vi "Calc Calculated Values.vi"(8 "error in":errorcluster, 10 "RT - Analysis Data in":T1={"RTController Data"={"State"=enum."Idle", "APU Setup Info"={"[[Sensor Info]]"=[], "[[Calibration Info]]"=[], "[[CMM Table 106]]"=[], "[[General APU Info]]"=[], "General APU Information"={"Run Count"=0}, "[[CMM Table 106B]] "=[]}, "Testing Select"=enum."Manual", "APU Select"="<Select>", "Subtests Array"=[], "Current Subtest&Step Indices"=[], "Fuel Pressure Regulator"=0.0, "Bleed-Fuel-ECS Controls"={"Fine_RC"=FALSE, "Fine_RO"=FALSE, "Coarse_RC"=FALSE, "Coarse_RO"=FALSE, "Bleed-Fine-Knob"=0.0, "Bleed-Coarse-Knob"=0.0}, "ECS Demand Cluster"={"02.06.9265.02"=4.0}, "APU & ECU Controls"={"02.00.9485.00"=FALSE, "02.01.9485.03"=FALSE, "02.01.9485.00"=FALSE, "02.01.9485.01"=FALSE, "02.00.9485.01"=FALSE, "02.00.9485.02"=FALSE, "02.00.9485.03"=FALSE, "02.00.9485.04"=FALSE, "02.00.9485.05"=FALSE, "02.01.9485.06"=FALSE, "02.00.9485.07"=FALSE, "00.04.9265.03"=FALSE}}, "Analyzed Data Sets"=[], "Current Vals"={"Post-Analysis Data"={"Calibrated Data"={"00-00-9205 Calib"=[], "00-01-9205 Calib"=[], "01-00-9213 Calib"=[], "01-01-9213 Calib"=[], "01-02-9213 Calib"=[], "02-02-9219 Calib"=[], "02-03-9227 Calib"=[], "00-02-9234 Calib"=[], "00-03-9402 Calib"=[], "02-05-9205 Calib"=[], "02-04-9871 2DArray"=[]}, "Calculated Data"={"C.00"=0.0, "C.01"=0.0, "C.02"=0.0, "C.03"=0.0, "C.04"=0.0, "C.05"=0.0, "C.06"=0.0, "C.07"=0.0, "C.08"=0.0, "C.09"=0.0, "C.10"=0.0, "C.11"=0.0, "C.12"=0.0, "C.13"=0.0, "C.14"=0.0, "C.15"=0.0, "C.16"=0.0, "C.17"=0.0, "C.18"=0.0, "C.19"=0.0, "C.20"=0.0, "C.21"=0.0, "C.22"=0.0, "C.23"=0.0, "C.24"=0.0, "C.25"=0.0, "C.26"=0.0, "C.27"=0.0, "C.28"=0.0, "C.29"=0.0, "C.30"=0.0, "C.31"=0.0, "C.32"=0.0, "C.33"=0.0, "C.34"=0.0, "C.35"=0.0, "C.36"=0.0, "C.37"=0.0, "C.38"=0.0, "C.39"=0.0, "C.40"=0.0, "C.41"=0.0, "C.42"=0.0, "C.43"=0.0, "C.44"=0.0, "C.45"=0.0, "C.46"=0.0, "C.47"=0.0, "C.48"=0.0, "C.49"=0.0, "C.50"=0.0, "C.51"=0.0, "C.52"=0.0, "C.53"=0.0, "C.54"=0.0, "C.56"=0.0}, "Indicator Data"={"00-02-9234 Power Spectras"=[], "00-02-9234 Peak Vel (in/sec)"=[], "Interactive Mode Vals"=[]}}, "Parsed Data Arrays"={"[Parsed Tags]"=[], "[VData out]"=[], "[Whole Tags]"=[]}}, "Samples/Sec"=0.0, "User Input Vals"=[], "Watchdogs"=[], "Interactive Data"={"Confirm Pressed"=FALSE, "Stored Vals"=[]}, "Accel Sensistivity"=[0.0, 0.0, 0.0], "Cutoff Frequncies"=[{"LP Passband"=0.0, "HP Stopband"=0.0, "LP Stopband"=0.0, "HP Passband"=0.0}, {"LP Passband"=0.0, "HP Stopband"=0.0, "LP Stopband"=0.0, "HP Passband"=0.0}, {"LP Passband"=0.0, "HP Stopband"=0.0, "LP Stopband"=0.0, "HP Passband"=0.0}], "Test Information"={"APU Part Number:"="", "Model:"="", "Serial Number:"="", "Customer:"="", "Work Order:"="", "Repair Level:"=""}} {"Cutoff Frequncies"."HP Passband" min=1.0 step=1.0 format="%#.4f"; "Cutoff Frequncies"."LP Stopband" min=1.0 step=1.0 format="%#.4f"; "Cutoff Frequncies"."HP Stopband" min=1.0 step=1.0 format="%#.4f"; "Cutoff Frequncies"."LP Passband" min=1.0 step=1.0 format="%#.4f"; "RTController Data"."ECS Demand Cluster"."02.06.9265.02" min=0.5 max=9.75 step=0.25 scale=0.5..9.75; "RTController Data"."Bleed-Fuel-ECS Controls"."Bleed-Coarse-Knob" min=0.0 max=1.0 step=0.001 scale=0.0..1.0; "RTController Data"."Bleed-Fuel-ECS Controls"."Bleed-Fine-Knob" min=0.0 max=1.0 step=0.001 scale=0.0..1.0; "RTController Data"."Fuel Pressure Regulator" min=0.0 max=100.0 step=0.25 scale=4.0..20.0}, 11 "[Params with Vals]":T23[](array[typedef])) -> (0 "error out":errorcluster, 3 "Calculated Values out":T16)   [LabVIEW 2018, in "RT - Analysis.lvlib"]
doc: "Performs all calculations to get the calculated values. Default output for a calculated value without an assigned calculation is NaN."
uses:
  RT - Analysis.lvlib
  Private Controls/Param Val Cluster.ctl
  Top Level/Shared Controls/Calculated Data.ctl
  Private Controls/RT-Analysis Data.ctl
  Private Controls/RTController Data.ctl
  Top Level/Shared Controls/cRIO State.ctl
  Top Level/Shared Controls/APU Setup File.ctl
  Modules/File IO/Public Controls/General APU Info.ctl
  Modules/Controller (Host)/Public Controls/Testing Select.ctl
  Modules/Controller (Host)/Public Controls/APU Select.ctl
  Modules/Testing UI 1/Public Controls/Fuel Pressure Regulator.ctl
  Modules/Testing UI 1/Public Controls/Bleed-Fuel-ECS Controls.ctl
  Modules/Testing UI 1/Public Controls/ECS Demand Controls.ctl
  Modules/Testing UI 1/Private Controls/APU & ECU Controls.ctl
  Top Level/Shared Controls/Analyzed Data Sets.ctl
  Top Level/Shared Controls/All Data Cluster.ctl
  Top Level/Shared Controls/Acq Data.ctl
  Top Level/Shared Controls/Post-Analysis Data.ctl
  Private Controls/Parsed Data Arrays.ctl
  Top Level/Shared Controls/Parsed Tag Cluster.ctl
  Private Controls/Watchdog Settings.ctl
  Private Controls/Interactive Data.ctl
  Modules/Testing UI 3/Private Controls/Cutoff Frequency.ctl
  Modules/Controller (Host)/Public Controls/Test Information.ctl
  <vilib>/Analysis/baseanly.llb/Mean (DBL).vi
  <vilib>/dlg_ctls.llb/Space Constant.vi
  Top Level/Shared VIs/Val Change Checker.vi
  <userlib>/_OpenG.lib/array/array.llb/Index Array Elements__ogtk.vi
  <userlib>/_OpenG.lib/array/array.llb/Index 1D Array Elements (Variant)__ogtk.vi
  <userlib>/_OpenG.lib/array/array.llb/Reorder 1D Array2 (DBL)__ogtk.vi
  <vilib>/Analysis/NI_AALBase.lvlib
  RT - Error Handler/RT - Error Handler.lvlib
  Modules/Controller (Host)/Controller (Host).lvlib
  Modules/Testing UI 1/Testing UI 1.lvlib
  Modules/File IO/File IO.lvlib
  Modules/Testing UI 3/Testing UI 3.lvlib
panel:
  # "Test Information:"
  # "Highpass Cutoff Frequency"
  # "Lowpass Cutoff Frequency"
  # "GTCP331-200ER Control Panel Discrete Input Panel"
  # "Bleed Load Controls"
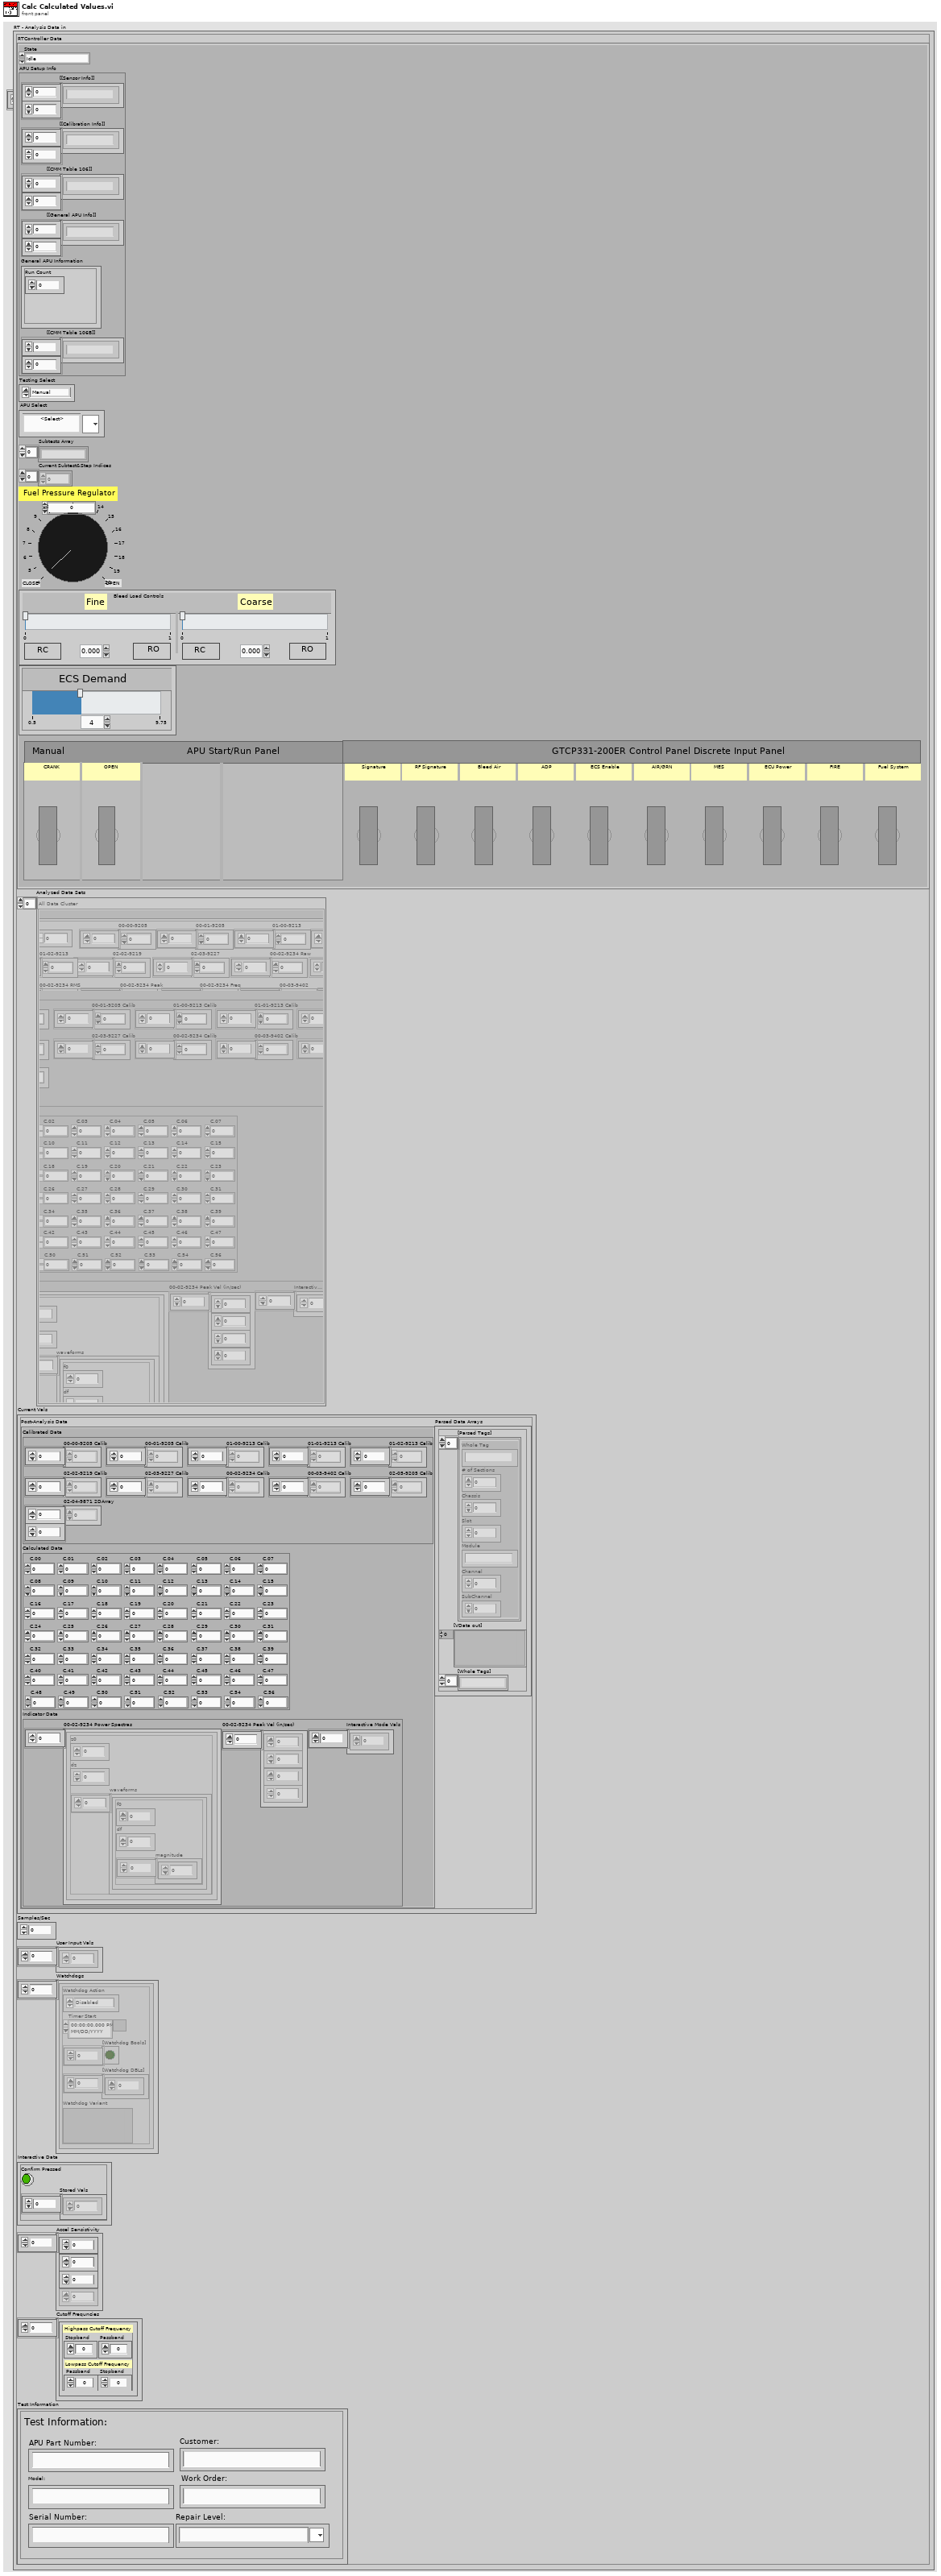
[diagram p1: front panel]
types:
  T1 = typedef "RT - Analysis.lvlib/RT-Analysis Data.ctl" = cluster{"RTController Data":T2, "Analyzed Data Sets":T12, "Current Vals":cluster{"Post-Analysis Data":T15, "Parsed Data Arrays":T17}, "Samples/Sec":dbl, "User Input Vals":dbl[], "Watchdogs":T19[], "Interactive Data":T20, "Accel Sensistivity":dbl[], "Cutoff Frequncies":T21[], "Test Information":T22}
  T2 = typedef "RT - Analysis.lvlib/RTController Data.ctl" = cluster{"State":T3, "APU Setup Info":T4, "Testing Select":T6, "APU Select":T7, "Subtests Array":string[], "Current Subtest&Step Indices":i32[], "Fuel Pressure Regulator":T8, "Bleed-Fuel-ECS Controls":T9, "ECS Demand Cluster":T10, "APU & ECU Controls":T11}
  T3 = typedef "cRIO State.ctl" = enum16{"Waiting for Cal Info", "Idle", "Calibration", "Testing"}
  T4 = typedef "APU Setup File.ctl" = cluster{"[[Sensor Info]]":string[][], "[[Calibration Info]]":string[][], "[[CMM Table 106]]":string[][], "[[General APU Info]]":string[][], "General APU Information":T5, "[[CMM Table 106B]] ":string[][]}
  T5 = typedef "File IO.lvlib/General APU Info.ctl" = cluster{"Run Count":u64}
  T6 = typedef "Controller (Host).lvlib/Testing Select.ctl" = enum16{"Manual", "Interactive", "Automatic"}
  T7 = typedef "Controller (Host).lvlib/APU Select.ctl" = string
  T8 = typedef "Testing UI 1.lvlib/Fuel Pressure Regulator.ctl" = dbl
  T9 = typedef "Testing UI 1.lvlib/Bleed-Fuel-ECS Controls.ctl" = cluster{"Fine_RC":bool, "Fine_RO":bool, "Coarse_RC":bool, "Coarse_RO":bool, "Bleed-Fine-Knob":dbl, "Bleed-Coarse-Knob":dbl}
  T10 = typedef "Testing UI 1.lvlib/ECS Demand Controls.ctl" = cluster{"02.06.9265.02":dbl}
  T11 = typedef "Testing UI 1.lvlib/APU & ECU Controls.ctl" = cluster{"02.00.9485.00":bool, "02.01.9485.03":bool, "02.01.9485.00":bool, "02.01.9485.01":bool, "02.00.9485.01":bool, "02.00.9485.02":bool, "02.00.9485.03":bool, "02.00.9485.04":bool, "02.00.9485.05":bool, "02.01.9485.06":bool, "02.00.9485.07":bool, "00.04.9265.03":bool}
  T12 = typedef "Analyzed Data Sets.ctl" = T13[]
  T13 = typedef "All Data Cluster.ctl" = cluster{"Acq Data":T14, "Post-Analysis Data":T15}
  T14 = typedef "Acq Data.ctl" = cluster{"Timestamp":timestamp, "Acq Period (ms)":i64, "00-00-9205":dbl[], "00-01-9205":dbl[], "01-00-9213":dbl[], "01-01-9213":dbl[], "01-02-9213":dbl[], "02-02-9219":dbl[], "02-03-9227":dbl[], "00-02-9234 Raw":dbl[], "00-02-9234 DC":dbl[], "00-02-9234 RMS":dbl[], "00-02-9234 Peak":dbl[], "00-02-9234 Freq":dbl[], "00-03-9402":dbl[], "02-05-9205":dbl[], "02-04-9871":dbl[]}
  T15 = typedef "Post-Analysis Data.ctl" = cluster{"Calibrated Data":cluster{"00-00-9205 Calib":dbl[], "00-01-9205 Calib":dbl[], "01-00-9213 Calib":dbl[], "01-01-9213 Calib":dbl[], "01-02-9213 Calib":dbl[], "02-02-9219 Calib":dbl[], "02-03-9227 Calib":dbl[], "00-02-9234 Calib":dbl[], "00-03-9402 Calib":dbl[], "02-05-9205 Calib":dbl[], "02-04-9871 2DArray":dbl[][]}, "Calculated Data":T16, "Indicator Data":cluster{"00-02-9234 Power Spectras":cluster{"z0":dbl, "dz":dbl, "waveforms":cluster{"f0":dbl, "df":dbl, "magnitude":dbl[]}[]}[], "00-02-9234 Peak Vel (in/sec)":dbl[], "Interactive Mode Vals":dbl[]}}
  T16 = typedef "Calculated Data.ctl" = cluster{"C.00":dbl, "C.01":dbl, "C.02":dbl, "C.03":dbl, "C.04":dbl, "C.05":dbl, "C.06":dbl, "C.07":dbl, "C.08":dbl, "C.09":dbl, "C.10":dbl, "C.11":dbl, "C.12":dbl, "C.13":dbl, "C.14":dbl, "C.15":dbl, "C.16":dbl, "C.17":dbl, "C.18":dbl, "C.19":dbl, "C.20":dbl, "C.21":dbl, "C.22":dbl, "C.23":dbl, "C.24":dbl, "C.25":dbl, "C.26":dbl, "C.27":dbl, "C.28":dbl, "C.29":dbl, "C.30":dbl, "C.31":dbl, "C.32":dbl, "C.33":dbl, "C.34":dbl, "C.35":dbl, "C.36":dbl, "C.37":dbl, "C.38":dbl, "C.39":dbl, "C.40":dbl, "C.41":dbl, "C.42":dbl, "C.43":dbl, "C.44":dbl, "C.45":dbl, "C.46":dbl, "C.47":dbl, "C.48":dbl, "C.49":dbl, "C.50":dbl, "C.51":dbl, "C.52":dbl, "C.53":dbl, "C.54":dbl, "C.56":dbl}
  T17 = typedef "RT - Analysis.lvlib/Parsed Data Arrays.ctl" = cluster{"[Parsed Tags]":T18[], "[VData out]":variant[], "[Whole Tags]":string[]}
  T18 = typedef "Parsed Tag Cluster.ctl" = cluster{"Whole Tag":string, "# of Sections":u8, "Chassis":u8, "Slot":u8, "Module":string, "Channel":u8, "SubChannel":u8}
  T19 = typedef "RT - Analysis.lvlib/Watchdog Settings.ctl" = cluster{"Watchdog Action":enum16{"Disabled", "Timer - Change Sample Rate", "RPM Thresh - Insert Other", "RPM Thresh - Check POPD", "RPM Thresh - StartStop Logging"}, "Timer Start":timestamp, "[Watchdog Bools]":bool[], "[Watchdog DBLs]":dbl[], "Watchdog Variant":variant}
  T20 = typedef "RT - Analysis.lvlib/Interactive Data.ctl" = cluster{"Confirm Pressed":bool, "Stored Vals":dbl[]}
  T21 = typedef "Testing UI 3.lvlib/Cutoff Frequency.ctl" = cluster{"LP Passband":dbl, "HP Stopband":dbl, "LP Stopband":dbl, "HP Passband":dbl}
  T22 = typedef "Controller (Host).lvlib/Test Information.ctl" = cluster{"APU Part Number:":string, "Model:":string, "Serial Number:":string, "Customer:":string, "Work Order:":string, "Repair Level:":string}
  T23 = typedef "RT - Analysis.lvlib/Param Val Cluster.ctl" = cluster{"Param":string, "Value":variant}
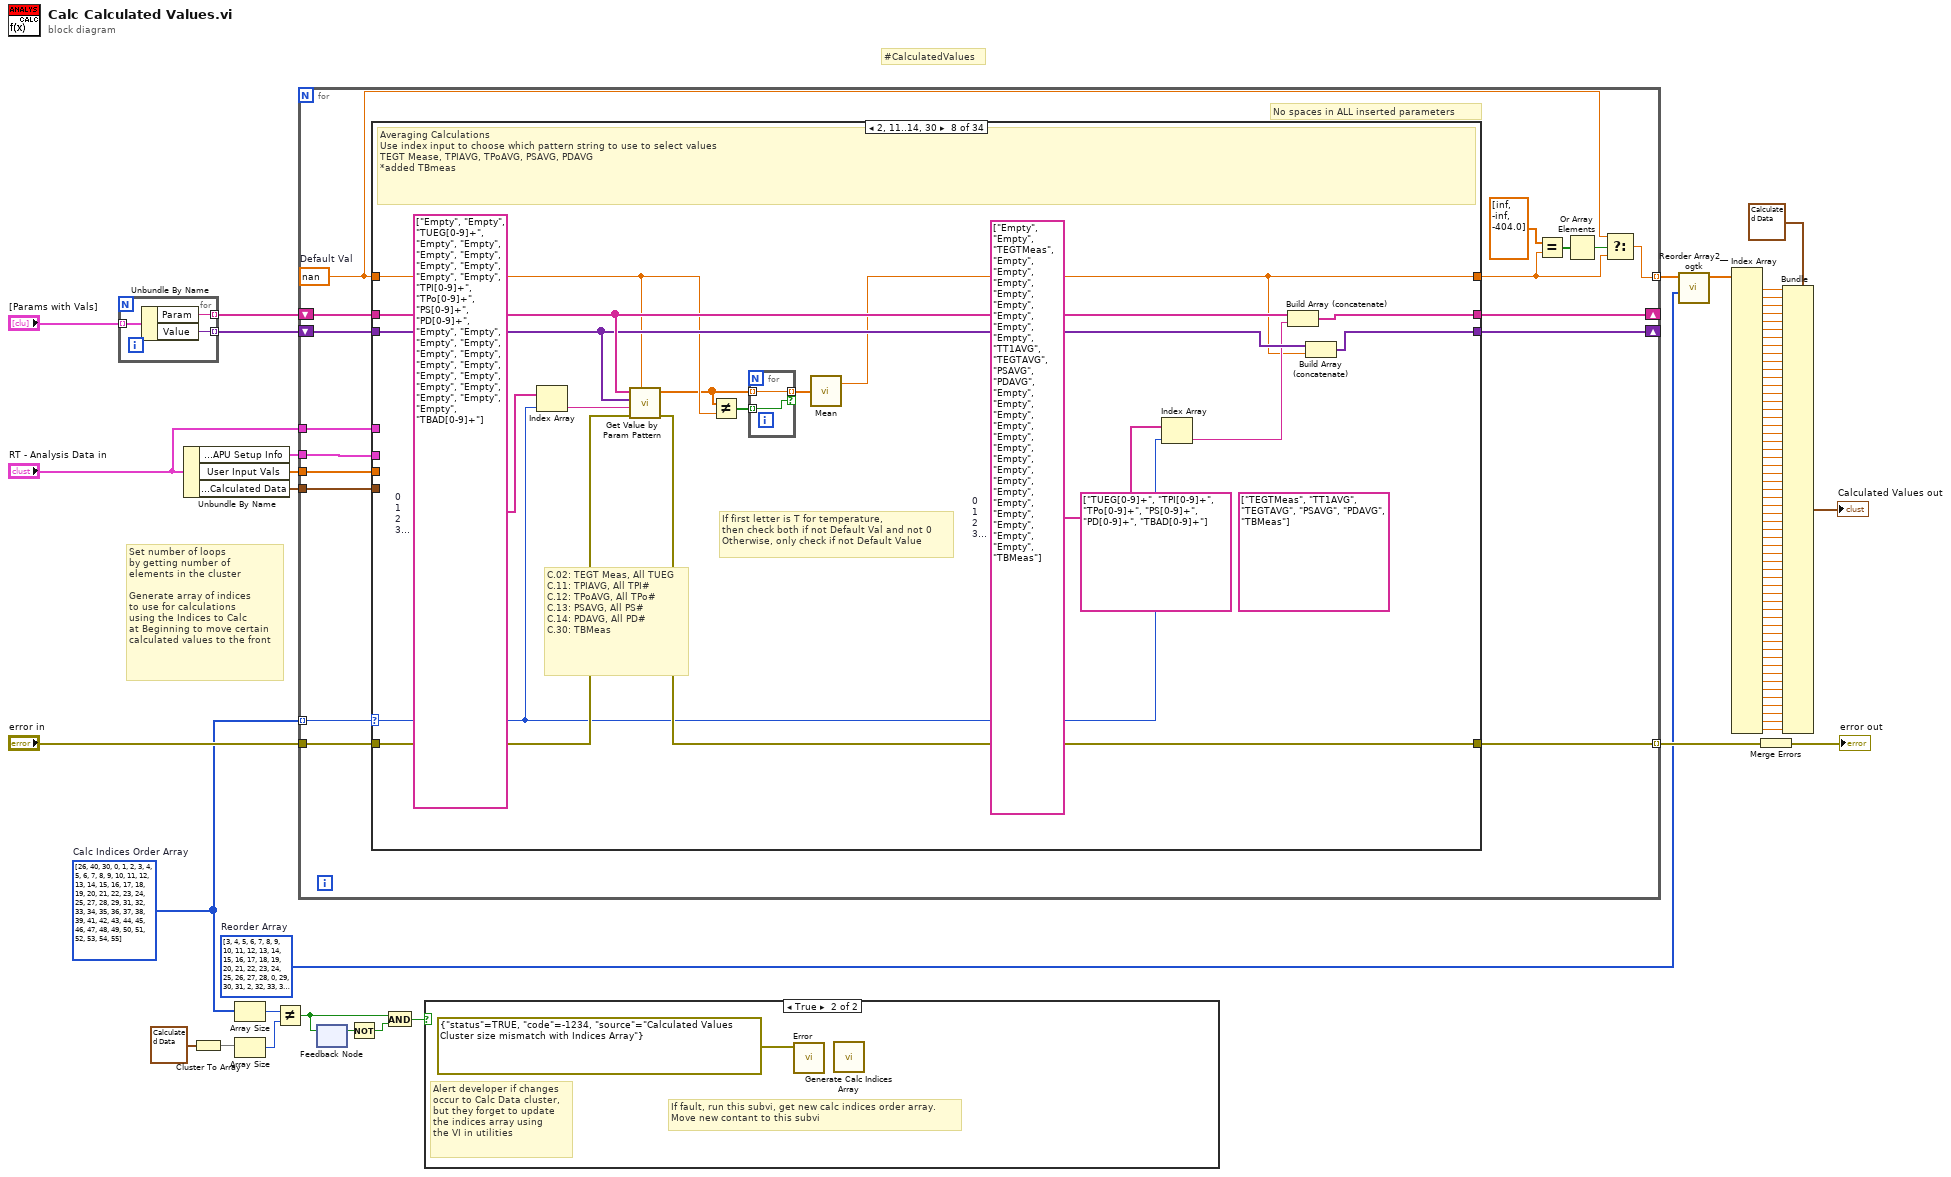
[diagram p0: block diagram]
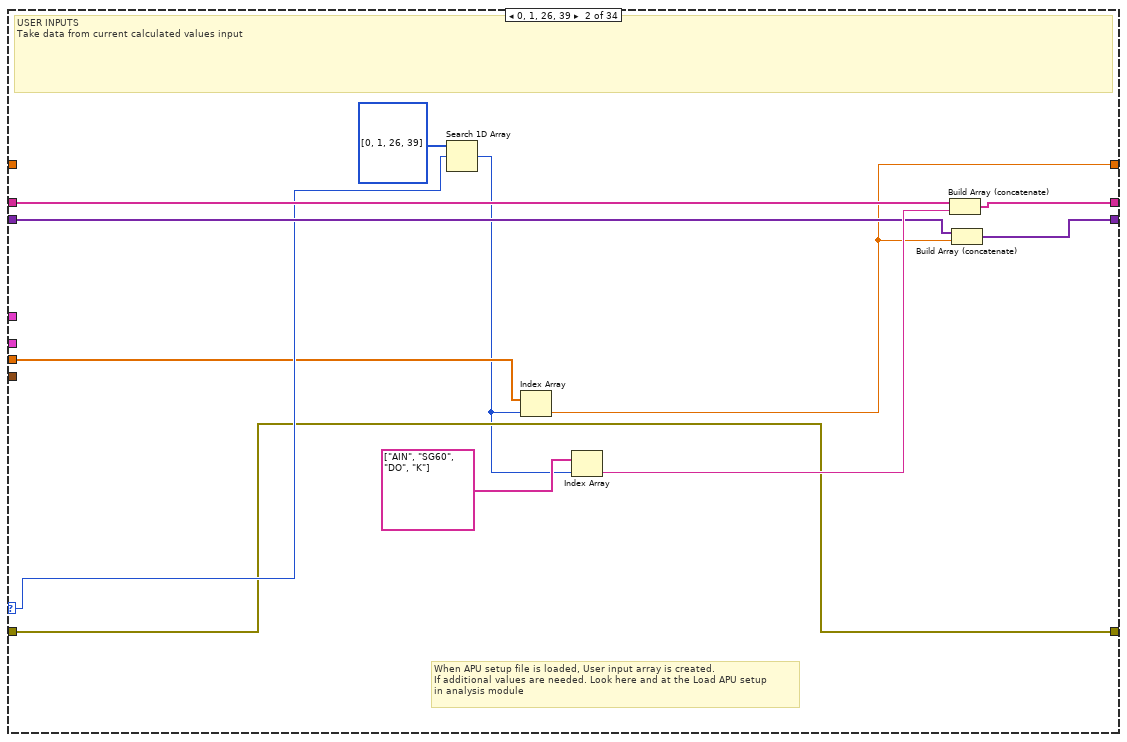
[diagram p4: hidden frame]
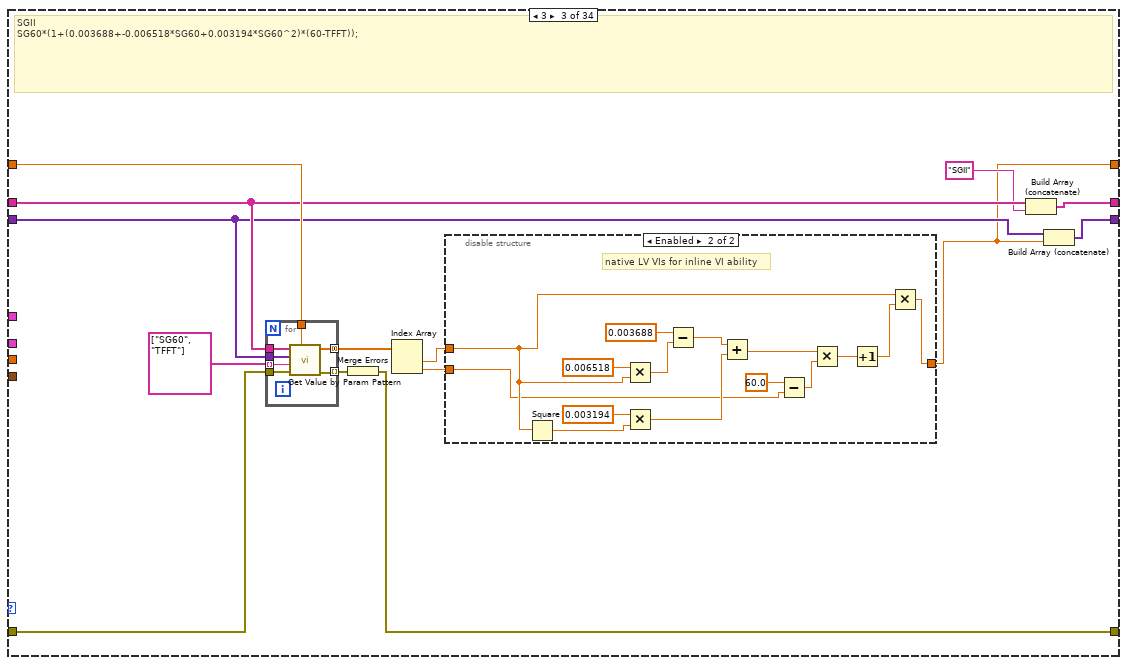
[diagram p5: hidden frame]
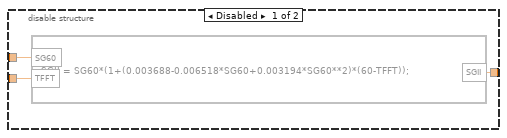
[diagram p6: hidden frame]
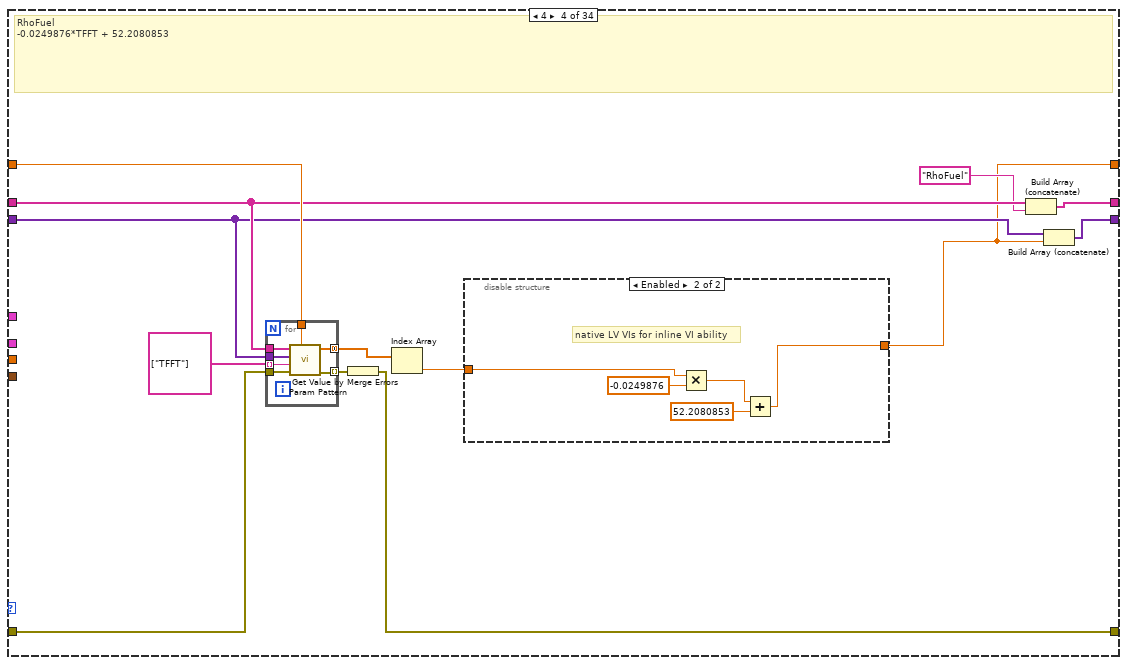
[diagram p7: hidden frame]
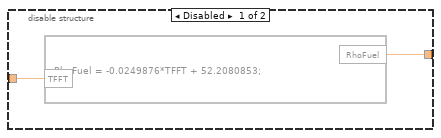
[diagram p8: hidden frame]
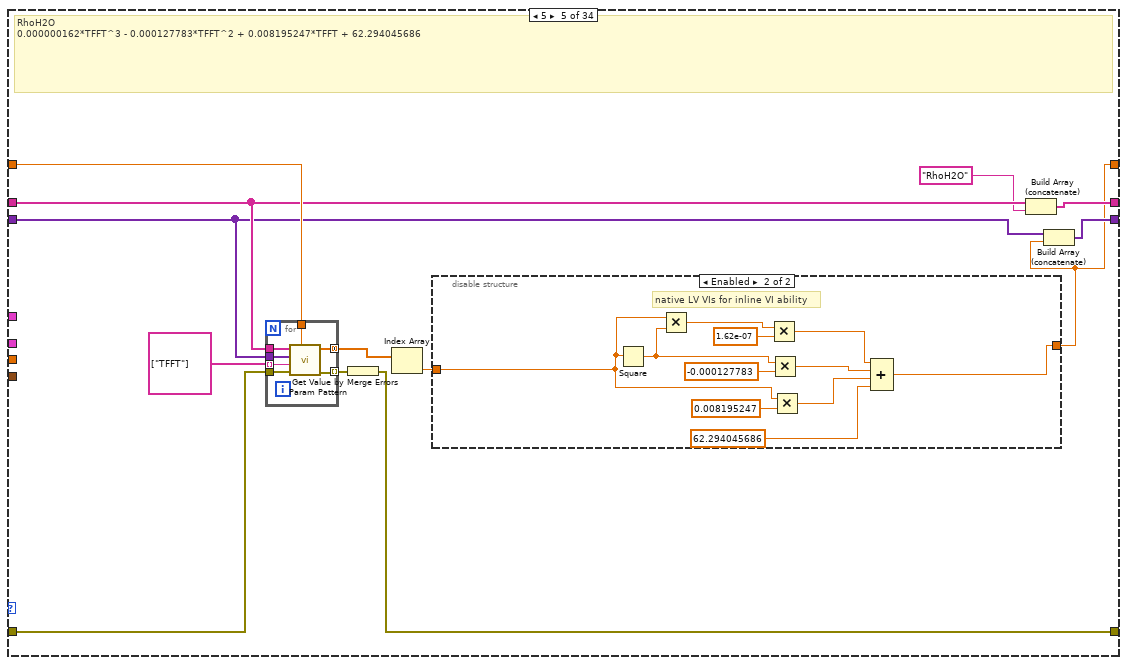
[diagram p9: hidden frame]
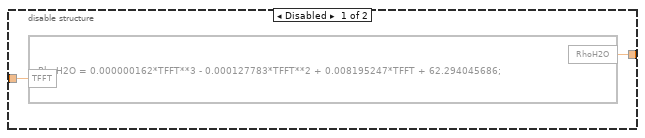
[diagram p10: hidden frame]
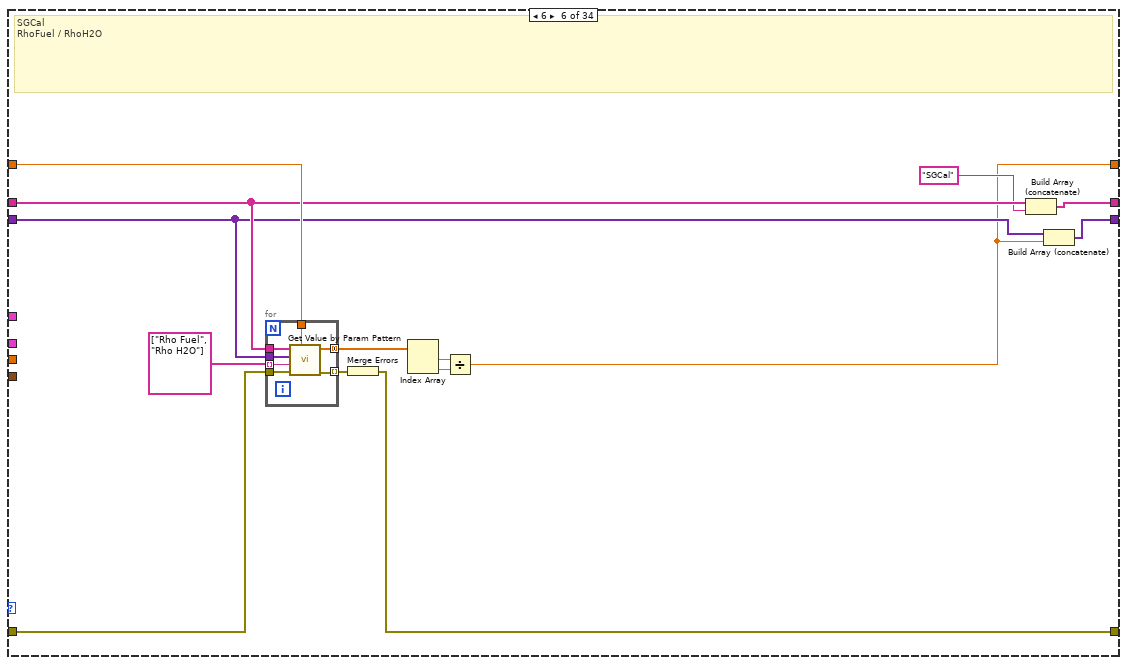
[diagram p11: hidden frame]
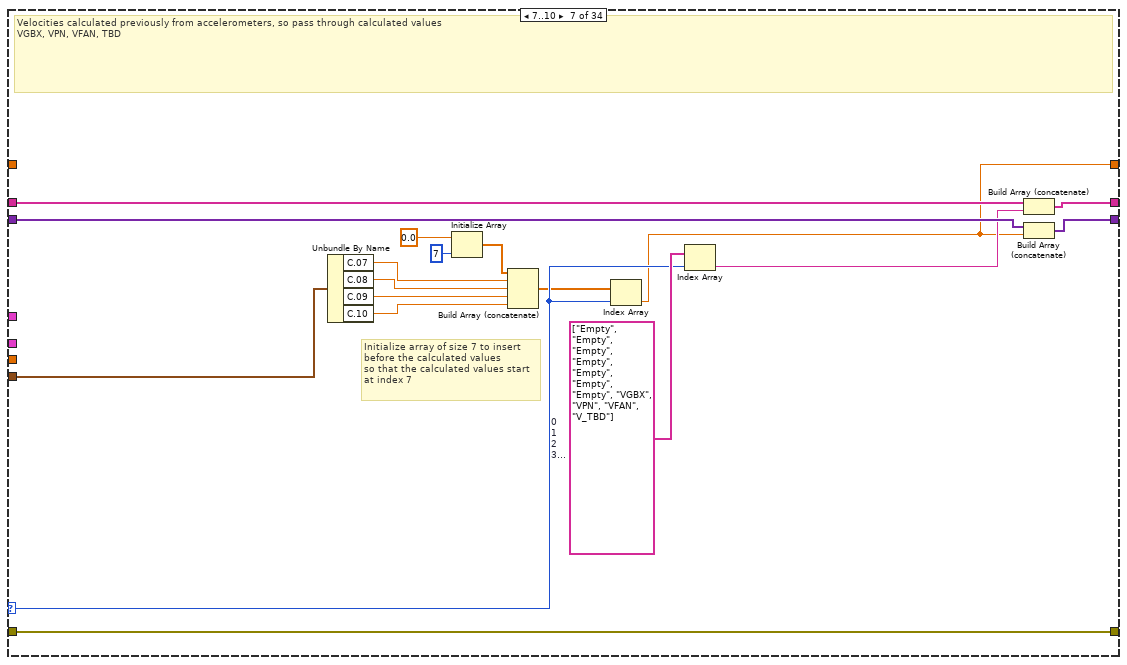
[diagram p12: hidden frame]
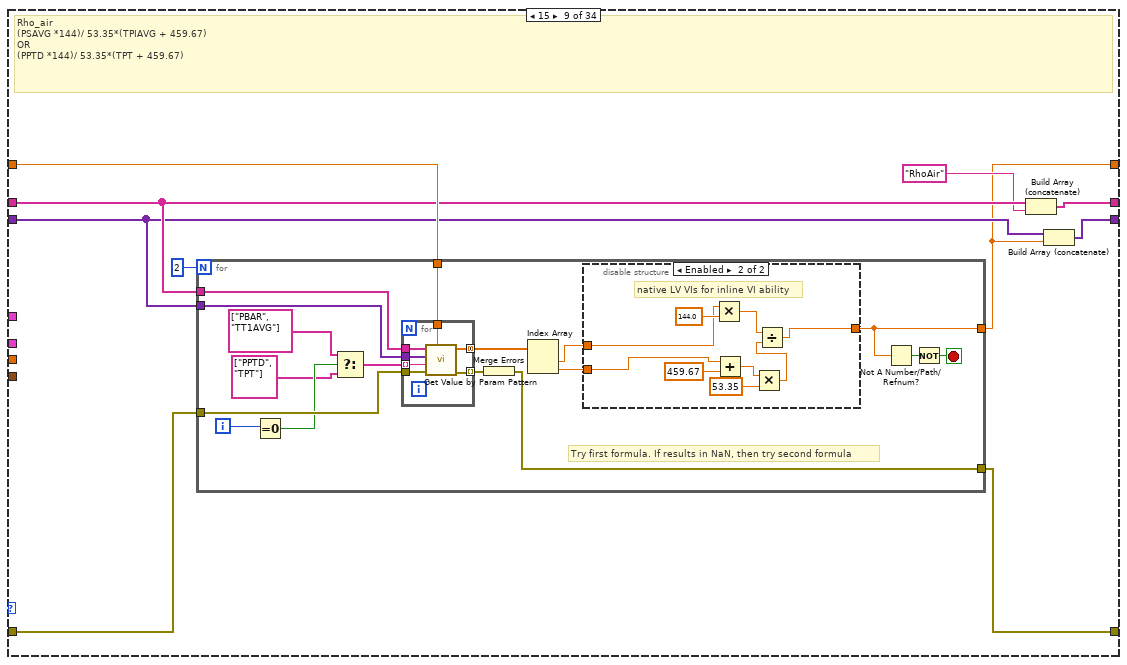
[diagram p13: hidden frame]
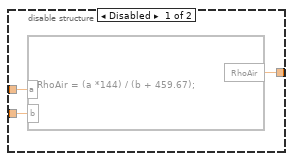
[diagram p14: hidden frame]
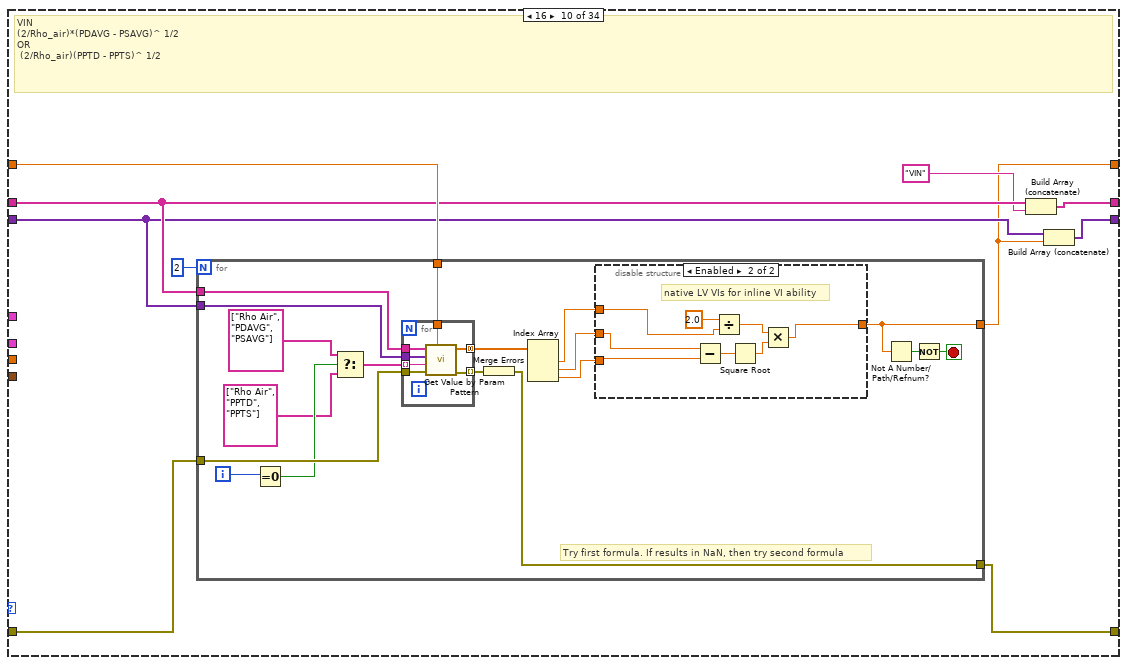
[diagram p15: hidden frame]
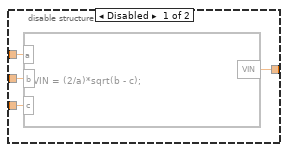
[diagram p16: hidden frame]
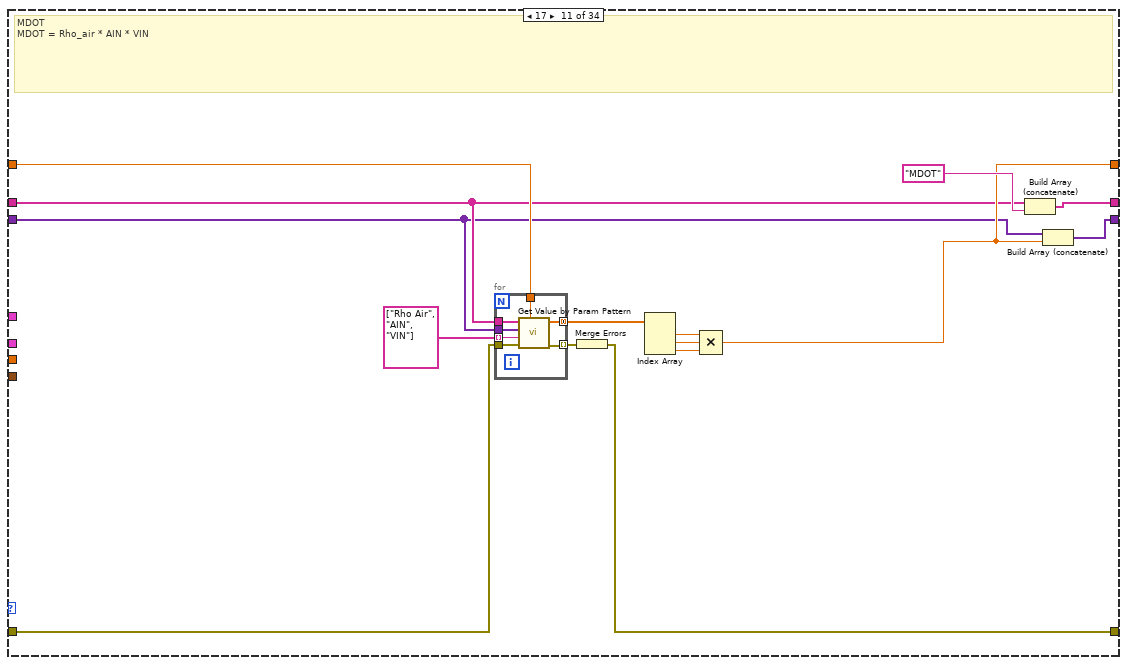
[diagram p17: hidden frame]
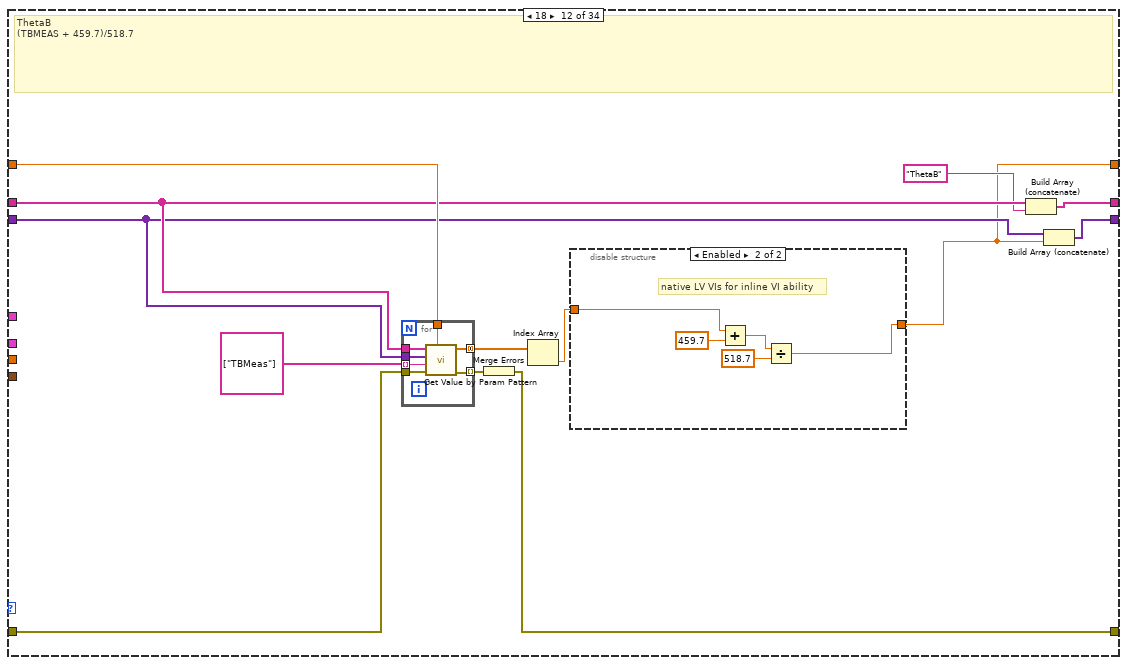
[diagram p18: hidden frame]
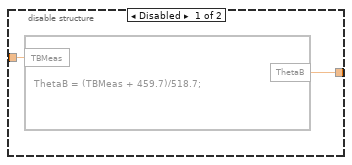
[diagram p19: hidden frame]
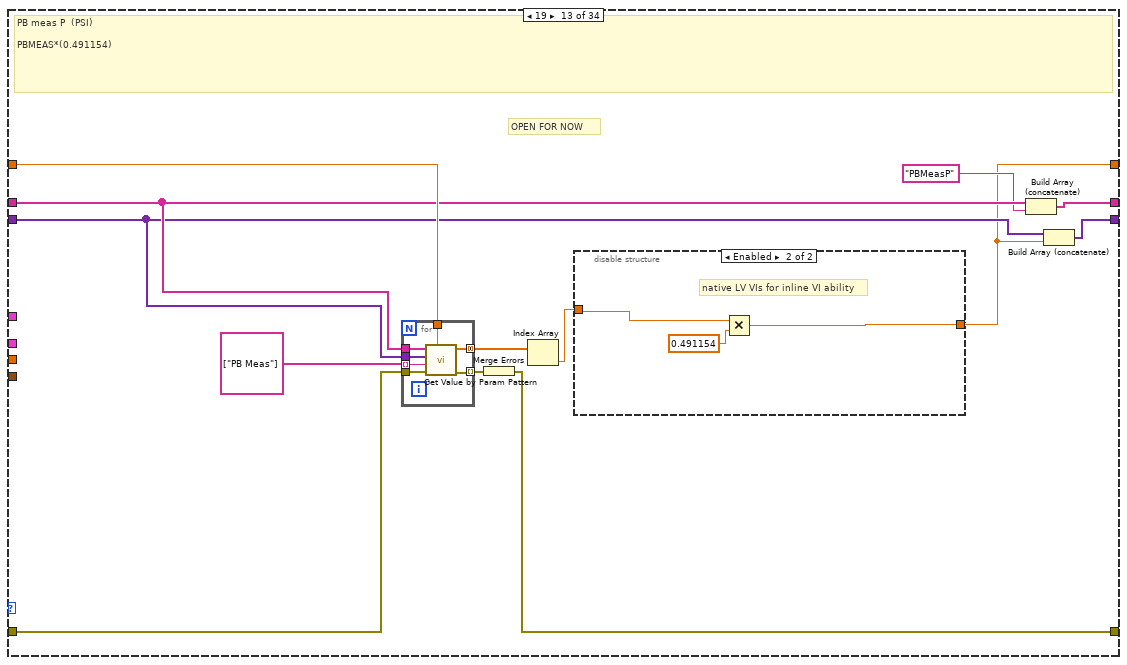
[diagram p20: hidden frame]
diagram:
  w2 = i32[] [3, 4, 5, 6, 7, 8, 9, 10, 11, 12, 13, 14, 15, 16, 17, 18, 19, 20, 21, 22, 23, 24, 25, 26, 27, 28, 0, 29, 30, 31, 2, 32, 33, 34, 35, 36, 37, 38, 39, 40, 1, 41, 42, 43, 44, 45, 46, 47, 48, 49, 50, 51, 52, 53, 54, 55]  # Reorder Array
  w3 = i32[] [26, 40, 30, 0, 1, 2, 3, 4, 5, 6, 7, 8, 9, 10, 11, 12, 13, 14, 15, 16, 17, 18, 19, 20, 21, 22, 23, 24, 25, 27, 28, 29, 31, 32, 33, 34, 35, 36, 37, 38, 39, 41, 42, 43, 44, 45, 46, 47, 48, 49, 50, 51, 52, 53, 54, 55]  # Calc Indices Order Array
  # "#CalculatedValues"
  # "Set number of loops\nby getting number of\nelements in the cluster\n\nGenerate array of indices\nto use for calculations\nusing the Indices to Calc\nat Beginning to move certain\ncalculated values to the front"
  n1 = for {
    tunnel: "[Params with Vals]" -> [w83] mode=indexing
    tunnel: [w82] -> w27 mode=indexing
    tunnel: [w81] -> w26 mode=indexing
    n2 = Unbundle By Name(w83) -> ("Param"=w82:string, "Value"=w81:variant)
  }
  n3 = Unbundle By Name("RT - Analysis Data in") -> ("RTController Data.APU Setup Info"=w7:T4, "User Input Vals"=w1:dbl[], "Current Vals.Post-Analysis Data.Calculated Data"=w23:T16)
  n4 = Cluster To Array(cluster=T16 {"C.00"=0.0, "C.01"=0.0, "C.02"=0.0, "C.03"=0.0, "C.04"=0.0, "C.05"=0.0, "C.06"=0.0, "C.07"=0.0, "C.08"=0.0, "C.09"=0.0, "C.10"=0.0, "C.11"=0.0, "C.12"=0.0, "C.13"=0.0, "C.14"=0.0, "C.15"=0.0, "C.16"=0.0, "C.17"=0.0, "C.18"=0.0, "C.19"=0.0, "C.20"=0.0, "C.21"=0.0, "C.22"=0.0, "C.23"=0.0, "C.24"=0.0, "C.25"=0.0, "C.26"=0.0, "C.27"=0.0, "C.28"=0.0, "C.29"=0.0, "C.30"=0.0, "C.31"=0.0, "C.32"=0.0, "C.33"=0.0, "C.34"=0.0, "C.35"=0.0, "C.36"=0.0, "C.37"=0.0, "C.38"=0.0, "C.39"=0.0, "C.40"=0.0, "C.41"=0.0, "C.42"=0.0, "C.43"=0.0, "C.44"=0.0, "C.45"=0.0, "C.46"=0.0, "C.47"=0.0, "C.48"=0.0, "C.49"=0.0, "C.50"=0.0, "C.51"=0.0, "C.52"=0.0, "C.53"=0.0, "C.54"=0.0, "C.56"=0.0} ("Current Vals.Post-Analysis Data.Calculated Data")) -> (array=w24:dbl[])
  n5 = Array Size(array=w3) -> (size(s)=w17:i32)
  n6 = Array Size(array=w24) -> (size(s)=w16:i32)
  n7 = Not Equal?(x=w17, y=w16) -> (x != y?=w20:bool)
  n8 = for {
    tunnel: [w89] -> w5 mode=indexing
    tunnel: [w98] -> w31 mode=indexing
    tunnel: "error in" -> [w97]
    shift-right: [w88] -> _
    shift-left: w27 -> [w100]
    shift-right: [w87] -> _
    shift-left: w26 -> [w99]
    tunnel: w23 -> [w96]
    tunnel: "RT - Analysis Data in" -> [w95]
    tunnel: w3 -> [w86] mode=indexing
    tunnel: w7 -> [w85]
    tunnel: w1 -> [w84]
    w91 = nan  # Default Val
    # "No spaces in ALL inserted parameters"
    n9 = case shown="2, 11..14, 30" w86 {
      selector: w86 -> [_ w109 _ _ _ _ w239 w259 _ _ _ _ _ _ _ _ _ _ _ _ w658 w690 _ _ _ _ _ _ _ _ _ _ _ _]
      tunnel: w100 -> [w102 w113 w128 w166 w193 w227 w251 w268 w278 w324 w369 w398 w425 w455 w484 w509 w536 w562 w609 w640 w662 w697 w725 w752 w780 w808 w836 w864 w907 w941 w975 w1014 w1044 w1072]
      tunnel: w99 -> [w101 w112 w126 w164 w191 w225 w250 w266 w276 w322 w368 w396 w423 w453 w482 w507 w534 w560 w607 w638 w661 w696 w726 w753 w781 w809 w837 w865 w908 w942 w976 w1015 w1045 w1073]
      tunnel: [w104 w110 w123 w161 w184 w216 w237 w262 w273 w319 w370 w393 w420 w445 w475 w504 w531 w557 w588 w629 w663 w691 w721 w748 w776 w804 w832 w860 w903 w937 w971 w1010 w1040 w1068] -> w90
      tunnel: w91 -> [w104 _ w130 w168 w195 w229 _ w258 w281 w327 w375 w400 w427 w440 w486 w511 w538 w564 w586 w642 w681 w708 w724 w751 w779 w807 w835 w863 w906 w940 w974 w1013 w1043 w1071]
      tunnel: [w103 w107 w129 w167 w194 w228 w254 w261 w279 w325 w376 w399 w426 w456 w485 w510 w537 w563 w610 w641 w680 w698 w722 w749 w777 w805 w833 w861 w904 w938 w972 w1011 w1041 w1069] -> w98
      tunnel: w97 -> [w103 w107 w119 w157 w185 w219 w254 w270 w280 w326 w377 w389 w415 w447 w476 w500 w527 w553 w596 w632 w682 w710 w723 w750 w778 w806 w834 w862 w905 w939 w973 w1012 w1042 w1070]
      tunnel: [w102 w111 w127 w165 w192 w226 w249 w267 w277 w323 w366 w397 w424 w454 w483 w508 w535 w561 w608 w639 w679 w707 w720 w747 w775 w803 w831 w859 w902 w936 w970 w1009 w1039 w1067] -> w88
      tunnel: [w101 w114 w125 w163 w190 w224 w248 w265 w275 w321 w367 w395 w422 w452 w481 w506 w533 w559 w606 w637 w678 w706 w719 w746 w774 w802 w830 w858 w901 w935 w969 w1008 w1038 w1066] -> w87
      tunnel: w96 -> [_ _ _ _ _ _ w253 _ _ _ _ _ _ _ _ _ _ _ _ _ _ _ _ _ _ _ _ _ _ _ _ _ _ _]
      tunnel: w95 -> [_ _ _ _ _ _ _ _ _ _ _ _ _ _ _ _ _ _ w601 _ w675 _ _ _ _ _ _ _ _ _ _ _ _ _]
      tunnel: w85 -> [_ _ _ _ _ _ _ _ _ _ _ _ _ _ _ _ _ _ _ _ _ _ _ _ _ _ _ _ _ _ _ _ _ _]
      tunnel: w84 -> [_ w106 _ _ _ _ _ _ _ _ _ _ _ _ _ _ _ _ _ _ _ _ _ _ _ _ _ _ _ _ _ _ _ _]
      frame -1, Default {
        # "Unhandled Calculated Value\nOutput DEFAULT value"
      }
      frame 0, 1, 26, 39 {
        # "When APU setup file is loaded, User input array is created. \nIf additional values are needed. Look here and at the Load APU setup \nin analysis module"
        # "USER INPUTS\nTake data from current calculated values input"
        n10 = Search 1D Array(1D array=i32[] [0, 1, 26, 39], element=w109) -> (index of element=w105:i32)  [unwired: 1 in]
        n11 = Index Array(array=w106, index=w105) -> (element=w110:dbl)
        n12 = Index Array(array=string[] ["AIN", "SG60", "DO", "K"], index=w105) -> (element=w115:string)
        n13 = Build Array (concatenate)(w113, w115) -> (w111:string[])
        n14 = Build Array (concatenate)(w112, w110) -> (w114:variant[])
      }
      frame 3 {
        # "SGII\nSG60*(1+(0.003688+-0.006518*SG60+0.003194*SG60^2)*(60-TFFT));"
        n15 = for {
          tunnel: w128 -> [w155]
          tunnel: w126 -> [w154]
          tunnel: w130 -> [w153]
          tunnel: w119 -> [w152]
          tunnel: [w151] -> w122 mode=indexing
          tunnel: [w150] -> w121 mode=concatenating
          tunnel: string[] ["SG60", "TFFT"] -> [w149] mode=indexing
          n16 = call "Get Value by Param Pattern.vi"("Default Val"=w153, "error in (no error)"=w152, "Pattern"=w149, "[Values]"=w154, "[Params]"=w155) -> ("error out"=w151:errorcluster, "[Values out]"=w150:dbl[])  [unwired: 5 in]
        }
        n17 = Merge Errors(w122) -> (w129:errorcluster)
        n18 = Index Array(array=w121) -> (element #1=w118:dbl, element #2=w117:dbl)  [unwired: 2 in]
        n19 = disable-structure shown="Enabled" {
          disable-tunnel: [w133 w134] -> w123
          disable-tunnel: w118 -> [w132 w136]
          disable-tunnel: w117 -> [w131 w135]
          frame Disabled {
            n20 = formula code="SGII = SG60*(1+(0.003688-0.006518*SG60+0.003194*SG60**2)*(60-TFFT));"("SG60"=w132, "TFFT"=w131) -> ("SGII"=w133:dbl)
          }
          frame Enabled {
            # "native LV VIs for inline VI ability"
            n21 = Square(x=w136) -> (x^2=w143:dbl)
            n22 = Multiply(x=0.006518, y=w136) -> (x*y=w138:dbl)
            n23 = Multiply(x=0.003194, y=w143) -> (x*y=w142:dbl)
            n24 = Subtract(x=0.003688, y=w138) -> (x-y=w140:dbl)
            n25 = Add(x=w140, y=w142) -> (x+y=w144:dbl)
            n26 = Subtract(x=60.0, y=w135) -> (x-y=w145:dbl)
            n27 = Multiply(x=w144, y=w145) -> (x*y=w147:dbl)
            n28 = Increment(x=w147) -> (x+1=w148:dbl)
            n29 = Multiply(x=w136, y=w148) -> (x*y=w134:dbl)
          }
        }
        n30 = Build Array (concatenate)(w128, "SGII" ("Param")) -> (w127:string[])
        n31 = Build Array (concatenate)(w126, w123) -> (w125:variant[])
      }
      frame 4 {
        # "RhoFuel\n-0.0249876*TFFT + 52.2080853"
        n32 = for {
          tunnel: w166 -> [w182]
          tunnel: w164 -> [w181]
          tunnel: w168 -> [w180]
          tunnel: w157 -> [w179]
          tunnel: [w178] -> w160 mode=indexing
          tunnel: [w177] -> w159 mode=concatenating
          tunnel: string[] ["TFFT"] -> [w176] mode=indexing
          n33 = call "Get Value by Param Pattern.vi"("Default Val"=w180, "error in (no error)"=w179, "Pattern"=w176, "[Values]"=w181, "[Params]"=w182) -> ("error out"=w178:errorcluster, "[Values out]"=w177:dbl[])  [unwired: 5 in]
        }
        n34 = Merge Errors(w160) -> (w167:errorcluster)
        n35 = Index Array(array=w159) -> (element=w156:dbl)  [unwired: 1 in]
        n36 = disable-structure shown="Enabled" {
          disable-tunnel: [w170 w171] -> w161
          disable-tunnel: w156 -> [w169 w172]
          frame Disabled {
            n37 = formula code="RhoFuel = -0.0249876*TFFT + 52.2080853;"("TFFT"=w169) -> ("RhoFuel"=w170:dbl)
          }
          frame Enabled {
            # "native LV VIs for inline VI ability"
            n38 = Multiply(x=w172, y=-0.0249876) -> (x*y=w173:dbl)
            n39 = Add(x=w173, y=52.2080853) -> (x+y=w171:dbl)
          }
        }
        n40 = Build Array (concatenate)(w166, "RhoFuel" ("Param")) -> (w165:string[])
        n41 = Build Array (concatenate)(w164, w161) -> (w163:variant[])
      }
      frame 5 {
        # "RhoH2O\n0.000000162*TFFT^3 - 0.000127783*TFFT^2 + 0.008195247*TFFT + 62.294045686"
        n42 = for {
          tunnel: w193 -> [w215]
          tunnel: w191 -> [w214]
          tunnel: w195 -> [w213]
          tunnel: w185 -> [w212]
          tunnel: [w211] -> w188 mode=indexing
          tunnel: [w210] -> w187 mode=concatenating
          tunnel: string[] ["TFFT"] -> [w209] mode=indexing
          n43 = call "Get Value by Param Pattern.vi"("Default Val"=w213, "error in (no error)"=w212, "Pattern"=w209, "[Values]"=w214, "[Params]"=w215) -> ("error out"=w211:errorcluster, "[Values out]"=w210:dbl[])  [unwired: 5 in]
        }
        n44 = Merge Errors(w188) -> (w194:errorcluster)
        n45 = Index Array(array=w187) -> (element=w183:dbl)  [unwired: 1 in]
        n46 = disable-structure shown="Enabled" {
          disable-tunnel: w183 -> [w197 w199]
          disable-tunnel: [w196 w198] -> w184
          frame Disabled {
            n47 = formula code="RhoH2O = 0.000000162*TFFT**3 - 0.000127783*TFFT**2 + 0.008195247*TFFT + 62.294045686;"("TFFT"=w197) -> ("RhoH2O"=w196:dbl)
          }
          frame Enabled {
            # "native LV VIs for inline VI ability"
            n48 = Square(x=w199) -> (x^2=w207:dbl)
            n49 = Multiply(x=w199, y=w207) -> (x*y=w208:dbl)
            n50 = Multiply(x=w208, y=1.62e-07) -> (x*y=w206:dbl)
            n51 = Multiply(x=w207, y=-0.000127783) -> (x*y=w205:dbl)
            n52 = Multiply(x=w199, y=0.008195247) -> (x*y=w204:dbl)
            n53 = Compound Arithmetic op=ADD(w206, w205, w204, 62.294045686 ("value")) -> (w198:dbl)
          }
        }
        n54 = Build Array (concatenate)(w193, "RhoH2O" ("Param")) -> (w192:string[])
        n55 = Build Array (concatenate)(w191, w184) -> (w190:variant[])
      }
      frame 6 {
        # "SGCal\nRhoFuel / RhoH2O"
        n56 = for {
          tunnel: w227 -> [w236]
          tunnel: w225 -> [w235]
          tunnel: w229 -> [w234]
          tunnel: w219 -> [w233]
          tunnel: [w232] -> w222 mode=indexing
          tunnel: [w231] -> w221 mode=concatenating
          tunnel: string[] ["Rho Fuel", "Rho H2O"] -> [w230] mode=indexing
          n57 = call "Get Value by Param Pattern.vi"("Default Val"=w234, "error in (no error)"=w233, "Pattern"=w230, "[Values]"=w235, "[Params]"=w236) -> ("error out"=w232:errorcluster, "[Values out]"=w231:dbl[])  [unwired: 5 in]
        }
        n58 = Merge Errors(w222) -> (w228:errorcluster)
        n59 = Index Array(array=w221) -> (element #1=w218:dbl, element #2=w217:dbl)  [unwired: 2 in]
        n60 = Divide(x=w218, y=w217) -> (x/y=w216:dbl)
        n61 = Build Array (concatenate)(w227, "SGCal" ("Param")) -> (w226:string[])
        n62 = Build Array (concatenate)(w225, w216) -> (w224:variant[])
      }
      frame 7..10 {
        w252 = string[] ["Empty", "Empty", "Empty", "Empty", "Empty", "Empty", "Empty", "VGBX", "VPN", "VFAN", "V_TBD"]  # 0 1 2 3 4 5 6 7 8 9 10
        # "Initialize array of size 7 to insert\nbefore the calculated values\nso that the calculated values start\nat index 7"
        # "Velocities calculated previously from accelerometers, so pass through calculated values\nVGBX, VPN, VFAN, TBD"
        n63 = Unbundle By Name(w253) -> ("C.07"=w246:dbl, "C.08"=w245:dbl, "C.09"=w244:dbl, "C.10"=w243:dbl)
        n64 = Initialize Array(0.0 ("element"), 7 ("dimension size")) -> (w240:dbl[])
        n65 = Build Array (concatenate)(w240, w246, w245, w244, w243) -> (w238:dbl[])
        n66 = Index Array(array=w238, index=w239) -> (element=w237:dbl)
        n67 = Index Array(array=w252, index=w239) -> (element=w247:string)
        n68 = Build Array (concatenate)(w251, w247) -> (w249:string[])
        n69 = Build Array (concatenate)(w250, w237) -> (w248:variant[])
      }
      frame 2, 11..14, 30 {
        (unwired) string[] ["TUEG[0-9]+", "TPI[0-9]+", "TPo[0-9]+", "PS[0-9]+", "PD[0-9]+", "TBAD[0-9]+"]
        (unwired) string[] ["TEGTMeas", "TT1AVG", "TEGTAVG", "PSAVG", "PDAVG", "TBMeas"]
        w264 = string[] ["Empty", "Empty", "TEGTMeas", "Empty", "Empty", "Empty", "Empty", "Empty", "Empty", "Empty", "Empty", "TT1AVG", "TEGTAVG", "PSAVG", "PDAVG", "Empty", "Empty", "Empty", "Empty", "Empty", "Empty", "Empty", "Empty", "Empty", "Empty", "Empty", "Empty", "Empty", "Empty", "Empty", "TBMeas"]  # 0 1 2 3 4 5 6 7 8 9 10 11 12 13 14 15 16 17 18 19 20 21 22 23 24 25 26 27 28 29 30
        w269 = string[] ["Empty", "Empty", "TUEG[0-9]+", "Empty", "Empty", "Empty", "Empty", "Empty", "Empty", "Empty", "Empty", "TPI[0-9]+", "TPo[0-9]+", "PS[0-9]+", "PD[0-9]+", "Empty", "Empty", "Empty", "Empty", "Empty", "Empty", "Empty", "Empty", "Empty", "Empty", "Empty", "Empty", "Empty", "Empty", "Empty", "TBAD[0-9]+"]  # 0 1 2 3 4 5 6 7 8 9 10 11 12 13 14 15 16 17 18 19 20 21 22 23 24 25 26 27 28 29 30
        # "If first letter is T for temperature,\nthen check both if not Default Val and not 0\nOtherwise, only check if not Default Value"
        # "C.02: TEGT Meas, All TUEG\nC.11: TPIAVG, All TPI#\nC.12: TPoAVG, All TPo#\nC.13: PSAVG, All PS#\nC.14: PDAVG, All PD#\nC.30: TBMeas"
        # "Averaging Calculations\nUse index input to choose which pattern string to use to select values\nTEGT Mease, TPIAVG, TPoAVG, PSAVG, PDAVG\n*added TBmeas"
        n70 = Index Array(array=w269, index=w259) -> (element=w257:string)
        n71 = call "Get Value by Param Pattern.vi"("Default Val"=w258, "error in (no error)"=w270, "Pattern"=w257, "[Values]"=w266, "[Params]"=w268) -> ("error out"=w261:errorcluster, "[Values out]"=w256:dbl[])  [unwired: 5 in]
        n72 = Not Equal?(x=w256, y=w258) -> (x != y?=w255:bool[])
        n73 = for {
          tunnel: w256 -> [w272] mode=indexing
          tunnel: [w272] -> w260 mode=indexing if=w271
          tunnel: w255 -> [w271] mode=indexing
        }
        n74 = call-poly <vilib>:"Mean.vi"("X"=w260) -> ("mean"=w262:dbl)  [unwired: 1 out]
        n75 = Index Array(array=w264, index=w259) -> (element=w263:string)
        n76 = Build Array (concatenate)(w268, w263) -> (w267:string[])
        n77 = Build Array (concatenate)(w266, w262) -> (w265:variant[])
      }
      frame 15 {
        # "Rho_air\n(PSAVG *144)/ 53.35*(TPIAVG + 459.67)\nOR\n(PPTD *144)/ 53.35*(TPT + 459.67)"
        n78 = for {
          N: 2 -> [_]
          tunnel: [w298] -> w273
          tunnel: w278 -> [w296]
          tunnel: w276 -> [w295]
          tunnel: w281 -> [w294]
          tunnel: w280 -> [w293]
          tunnel: [w292] -> w279
          i -> [w287]
          stop <- w297 stop-if-true
          # "Try first formula. If results in NaN, then try second formula"
          n79 = Equal To 0?(x=w287) -> (x = 0?=w285:bool)
          n80 = Select(t=string[] ["PBAR", "TT1AVG"], s=w285, f=string[] ["PPTD", "TPT"]) -> (s? t:f=w286:string[])
          n81 = for {
            tunnel: w296 -> [w318]
            tunnel: w295 -> [w317]
            tunnel: w294 -> [w316]
            tunnel: w293 -> [w315]
            tunnel: [w314] -> w291 mode=indexing
            tunnel: [w313] -> w290 mode=concatenating
            tunnel: w286 -> [w312] mode=indexing
            n82 = call "Get Value by Param Pattern.vi"("Default Val"=w316, "error in (no error)"=w315, "Pattern"=w312, "[Values]"=w317, "[Params]"=w318) -> ("error out"=w314:errorcluster, "[Values out]"=w313:dbl[])  [unwired: 5 in]
          }
          n83 = Merge Errors(w291) -> (w292:errorcluster)
          n84 = Index Array(array=w290) -> (element #1=w289:dbl, element #2=w288:dbl)  [unwired: 2 in]
          n85 = disable-structure shown="Enabled" {
            disable-tunnel: [w302 w306] -> w298
            disable-tunnel: w289 -> [w301 w308]
            disable-tunnel: w288 -> [w300 w307]
            frame Disabled {
              n86 = formula code="RhoAir = (a *144) / (b + 459.67);"("b"=w300, "a"=w301) -> ("RhoAir"=w302:dbl)
            }
            frame Enabled {
              # "native LV VIs for inline VI ability"
              n87 = Multiply(x=w308, y=144.0) -> (x*y=w309:dbl)
              n88 = Add(x=w307, y=459.67) -> (x+y=w305:dbl)
              n89 = Multiply(x=w305, y=53.35) -> (x*y=w304:dbl)
              n90 = Divide(x=w309, y=w304) -> (x/y=w306:dbl)
            }
          }
          n91 = Not A Number/Path/Refnum?(number/path/refnum=w298) -> (NaN/Path/Refnum?=w299:bool)
          n92 = Not(x=w299) -> (.not. x?=w297:bool)
        }
        n93 = Build Array (concatenate)(w278, "RhoAir" ("Param")) -> (w277:string[])
        n94 = Build Array (concatenate)(w276, w273) -> (w275:variant[])
      }
      frame 16 {
        # "VIN\n(2/Rho_air)*(PDAVG - PSAVG)^ 1/2\nOR\n (2/Rho_air)(PPTD - PPTS)^ 1/2"
        n95 = for {
          N: 2 -> [_]
          tunnel: [w329] -> w319
          tunnel: w324 -> [w344]
          tunnel: w322 -> [w343]
          tunnel: w327 -> [w342]
          tunnel: w326 -> [w341]
          tunnel: [w340] -> w325
          i -> [w335]
          stop <- w345 stop-if-true
          # "Try first formula. If results in NaN, then try second formula"
          n96 = Equal To 0?(x=w335) -> (x = 0?=w333:bool)
          n97 = Select(t=string[] ["Rho Air", "PDAVG", "PSAVG"], s=w333, f=string[] ["Rho Air", "PPTD", "PPTS"]) -> (s? t:f=w334:string[])
          n98 = for {
            tunnel: w344 -> [w365]
            tunnel: w343 -> [w364]
            tunnel: w342 -> [w363]
            tunnel: w341 -> [w362]
            tunnel: [w361] -> w339 mode=indexing
            tunnel: [w360] -> w338 mode=concatenating
            tunnel: w334 -> [w359] mode=indexing
            n99 = call "Get Value by Param Pattern.vi"("Default Val"=w363, "error in (no error)"=w362, "Pattern"=w359, "[Values]"=w364, "[Params]"=w365) -> ("error out"=w361:errorcluster, "[Values out]"=w360:dbl[])  [unwired: 5 in]
          }
          n100 = Merge Errors(w339) -> (w340:errorcluster)
          n101 = Index Array(array=w338) -> (element #1=w337:dbl, element #2=w336:dbl, element #3=w330:dbl)  [unwired: 3 in]
          n102 = disable-structure shown="Enabled" {
            disable-tunnel: w337 -> [w350 w354]
            disable-tunnel: w336 -> [w349 w353]
            disable-tunnel: w330 -> [w348 w352]
            disable-tunnel: [w347 w351] -> w329
            frame Disabled {
              n103 = formula code="VIN = (2/a)*sqrt(b - c);"("b"=w349, "a"=w350, "c"=w348) -> ("VIN"=w347:dbl)
            }
            frame Enabled {
              # "native LV VIs for inline VI ability"
              n104 = Subtract(x=w353, y=w352) -> (x-y=w358:dbl)
              n105 = Divide(x=2.0, y=w354) -> (x/y=w356:dbl)
              n106 = Square Root(x=w358) -> (sqrt(x)=w357:dbl)
              n107 = Multiply(x=w356, y=w357) -> (x*y=w351:dbl)
            }
          }
          n108 = Not A Number/Path/Refnum?(number/path/refnum=w329) -> (NaN/Path/Refnum?=w346:bool)
          n109 = Not(x=w346) -> (.not. x?=w345:bool)
        }
        n110 = Build Array (concatenate)(w324, "VIN" ("Param")) -> (w323:string[])
        n111 = Build Array (concatenate)(w322, w319) -> (w321:variant[])
      }
      frame 17 {
        # "MDOT\nMDOT = Rho_air * AIN * VIN"
        n112 = for {
          tunnel: w369 -> [w387]
          tunnel: w368 -> [w386]
          tunnel: w375 -> [w385]
          tunnel: w377 -> [w384]
          tunnel: [w383] -> w380 mode=indexing
          tunnel: [w382] -> w379 mode=concatenating
          tunnel: string[] ["Rho Air", "AIN", "VIN"] -> [w381] mode=indexing
          n113 = call "Get Value by Param Pattern.vi"("Default Val"=w385, "error in (no error)"=w384, "Pattern"=w381, "[Values]"=w386, "[Params]"=w387) -> ("error out"=w383:errorcluster, "[Values out]"=w382:dbl[])  [unwired: 5 in]
        }
        n114 = Merge Errors(w380) -> (w376:errorcluster)
        n115 = Index Array(array=w379) -> (element #1=w374:dbl, element #2=w373:dbl, element #3=w372:dbl)  [unwired: 3 in]
        n116 = Compound Arithmetic op=MULTIPLY(w374, w373, w372) -> (w370:dbl)
        n117 = Build Array (concatenate)(w369, "MDOT" ("Param")) -> (w366:string[])
        n118 = Build Array (concatenate)(w368, w370) -> (w367:variant[])
      }
      frame 18 {
        # "ThetaB\n(TBMEAS + 459.7)/518.7"
        n119 = for {
          tunnel: w398 -> [w414]
          tunnel: w396 -> [w413]
          tunnel: w400 -> [w412]
          tunnel: w389 -> [w411]
          tunnel: [w410] -> w392 mode=indexing
          tunnel: [w409] -> w391 mode=concatenating
          tunnel: string[] ["TBMeas"] -> [w408] mode=indexing
          n120 = call "Get Value by Param Pattern.vi"("Default Val"=w412, "error in (no error)"=w411, "Pattern"=w408, "[Values]"=w413, "[Params]"=w414) -> ("error out"=w410:errorcluster, "[Values out]"=w409:dbl[])  [unwired: 5 in]
        }
        n121 = Merge Errors(w392) -> (w399:errorcluster)
        n122 = Index Array(array=w391) -> (element=w388:dbl)  [unwired: 1 in]
        n123 = disable-structure shown="Enabled" {
          disable-tunnel: [w402 w403] -> w393
          disable-tunnel: w388 -> [w401 w404]
          frame Disabled {
            n124 = formula code="ThetaB = (TBMeas + 459.7)/518.7;"("TBMeas"=w401) -> ("ThetaB"=w402:dbl)
          }
          frame Enabled {
            # "native LV VIs for inline VI ability"
            n125 = Add(x=w404, y=459.7) -> (x+y=w406:dbl)
            n126 = Divide(x=w406, y=518.7) -> (x/y=w403:dbl)
          }
        }
        n127 = Build Array (concatenate)(w398, "ThetaB" ("Param")) -> (w397:string[])
        n128 = Build Array (concatenate)(w396, w393) -> (w395:variant[])
      }
      frame 19 {
        # "OPEN FOR NOW"
        # "PB meas P  (PSI)\n\nPBMEAS*(0.491154)"
        n129 = for {
          tunnel: w425 -> [w439]
          tunnel: w423 -> [w438]
          tunnel: w427 -> [w437]
          tunnel: w415 -> [w436]
          tunnel: [w435] -> w419 mode=indexing
          tunnel: [w434] -> w418 mode=concatenating
          tunnel: string[] ["PB Meas"] -> [w433] mode=indexing
          n130 = call "Get Value by Param Pattern.vi"("Default Val"=w437, "error in (no error)"=w436, "Pattern"=w433, "[Values]"=w438, "[Params]"=w439) -> ("error out"=w435:errorcluster, "[Values out]"=w434:dbl[])  [unwired: 5 in]
        }
        n131 = Merge Errors(w419) -> (w426:errorcluster)
        n132 = Index Array(array=w418) -> (element=w417:dbl)  [unwired: 1 in]
        n133 = disable-structure shown="Enabled" {
          disable-tunnel: [w429 w430] -> w420
          disable-tunnel: w417 -> [w428 w432]
          frame Disabled {
            n134 = formula code="DeltaPBCOR = PBMeas/(14.7/0.49109778);"("PBMeas"=w428) -> ("DeltaPBCOR"=w429:dbl)
          }
          frame Enabled {
            # "native LV VIs for inline VI ability"
            n135 = Multiply(x=w432, y=0.491154) -> (x*y=w430:dbl)
          }
        }
        n136 = Build Array (concatenate)(w425, "PBMeasP" ("Param")) -> (w424:string[])
        n137 = Build Array (concatenate)(w423, w420) -> (w422:variant[])
      }
      frame 20 {
        w441 = 0.1  # Threshold for PBMeas to ensure calculated value is accurate
        # "PBCOR\n((PBMEAS P) / ((Pbar*0.491154)/14.7))"
        n138 = for {
          tunnel: w455 -> [w473]
          tunnel: w453 -> [w472]
          tunnel: w440 -> [w471]
          tunnel: w447 -> [w470]
          tunnel: [w469] -> w450 mode=indexing
          tunnel: [w468] -> w449 mode=concatenating
          tunnel: string[] ["PBMeasP", "PBAR"] -> [w467] mode=indexing
          n139 = call "Get Value by Param Pattern.vi"("Default Val"=w471, "error in (no error)"=w470, "Pattern"=w467, "[Values]"=w472, "[Params]"=w473) -> ("error out"=w469:errorcluster, "[Values out]"=w468:dbl[])  [unwired: 5 in]
        }
        n140 = Merge Errors(w450) -> (w456:errorcluster)
        n141 = Index Array(array=w449) -> (element #1=w442:dbl, element #2=w446:dbl)  [unwired: 2 in]
        n142 = disable-structure shown="Enabled" {
          disable-tunnel: [w459 w464] -> w444
          disable-tunnel: w442 -> [w458 w463]
          disable-tunnel: w446 -> [w457 w462]
          frame Disabled {
            n143 = formula code="PBCOR = ((PBMeas*0.49109778)-14.7)/PAMB;\nDeltaB = ((PBMeas*0.49109778))/14.7;"("PBMeas"=w458, "PAMB"=w457) -> ("PBCOR"=w459:dbl)  [unwired: 1 out]
          }
          frame Enabled {
            # "native LV VIs for inline VI ability"
            n144 = Multiply(x=w462, y=0.491154) -> (x*y=w460:dbl)
            n145 = Divide(x=w460, y=14.7) -> (x/y=w465:dbl)
            n146 = Divide(x=w463, y=w465) -> (x/y=w464:dbl)
          }
        }
        n147 = Greater Or Equal?(x=w442, y=w441) -> (x >= y?=w443:bool)
        n148 = Build Array (concatenate)(w455, "PBCOR" ("Param")) -> (w454:string[])
        n149 = Select(t=w444, s=w443, f=w440) -> (s? t:f=w445:dbl)
        n150 = Build Array (concatenate)(w453, w445) -> (w452:variant[])
      }
      frame 21 {
        # "DeltaB\n((PBMeas P))/14.7;"
        n151 = for {
          tunnel: w484 -> [w498]
          tunnel: w482 -> [w497]
          tunnel: w486 -> [w496]
          tunnel: w476 -> [w495]
          tunnel: [w494] -> w479 mode=indexing
          tunnel: [w493] -> w478 mode=concatenating
          tunnel: string[] ["PBMeasP"] -> [w492] mode=indexing
          n152 = call "Get Value by Param Pattern.vi"("Default Val"=w496, "error in (no error)"=w495, "Pattern"=w492, "[Values]"=w497, "[Params]"=w498) -> ("error out"=w494:errorcluster, "[Values out]"=w493:dbl[])  [unwired: 5 in]
        }
        n153 = Merge Errors(w479) -> (w485:errorcluster)
        n154 = Index Array(array=w478) -> (element=w474:dbl)  [unwired: 1 in]
        n155 = disable-structure shown="Enabled" {
          disable-tunnel: [w488 w490] -> w475
          disable-tunnel: w474 -> [w487 w489]
          frame Disabled {
            n156 = formula code="DeltaB = ((PBMeas*0.49109778))/14.7;"("PBMeas"=w487) -> ("DeltaB"=w488:dbl)  [unwired: 1 out]
          }
          frame Enabled {
            # "native LV VIs for inline VI ability"
            n157 = Divide(x=w489, y=14.7) -> (x/y=w490:dbl)
          }
        }
        n158 = Build Array (concatenate)(w484, "DeltaB" ("Param")) -> (w483:string[])
        n159 = Build Array (concatenate)(w482, w475) -> (w481:variant[])
      }
      frame 22 {
        # "dPAMB\n(PBAR * 0.491154)/(14.7/))"
        n160 = for {
          tunnel: w509 -> [w525]
          tunnel: w507 -> [w524]
          tunnel: w511 -> [w523]
          tunnel: w500 -> [w522]
          tunnel: [w521] -> w503 mode=indexing
          tunnel: [w520] -> w502 mode=concatenating
          tunnel: string[] ["PBAR"] -> [w519] mode=indexing
          n161 = call "Get Value by Param Pattern.vi"("Default Val"=w523, "error in (no error)"=w522, "Pattern"=w519, "[Values]"=w524, "[Params]"=w525) -> ("error out"=w521:errorcluster, "[Values out]"=w520:dbl[])  [unwired: 5 in]
        }
        n162 = Merge Errors(w503) -> (w510:errorcluster)
        n163 = Index Array(array=w502) -> (element=w499:dbl)  [unwired: 1 in]
        n164 = disable-structure shown="Enabled" {
          disable-tunnel: [w513 w518] -> w504
          disable-tunnel: w499 -> [w512 w517]
          frame Disabled {
            n165 = formula code="DeltaPAMB = (PAMB)/(14.7/0.49109778);"("PAMB"=w512) -> ("DeltaPAMB"=w513:dbl)
          }
          frame Enabled {
            # "native LV VIs for inline VI ability"
            n166 = Multiply(x=w517, y=0.491154) -> (x*y=w515:dbl)
            n167 = Divide(x=w515, y=14.7 ("x")) -> (x/y=w518:dbl)
          }
        }
        n168 = Build Array (concatenate)(w509, "DeltaPAMB1" ("Param")) -> (w508:string[])
        n169 = Build Array (concatenate)(w507, w504) -> (w506:variant[])
      }
      frame 23 {
        # "Pamb P\n(PBAR*0.491154)"
        n170 = for {
          tunnel: w536 -> [w550]
          tunnel: w534 -> [w549]
          tunnel: w538 -> [w548]
          tunnel: w527 -> [w547]
          tunnel: [w546] -> w530 mode=indexing
          tunnel: [w545] -> w529 mode=concatenating
          tunnel: string[] ["PBAR"] -> [w544] mode=indexing
          n171 = call "Get Value by Param Pattern.vi"("Default Val"=w548, "error in (no error)"=w547, "Pattern"=w544, "[Values]"=w549, "[Params]"=w550) -> ("error out"=w546:errorcluster, "[Values out]"=w545:dbl[])  [unwired: 5 in]
        }
        n172 = Merge Errors(w530) -> (w537:errorcluster)
        n173 = Index Array(array=w529) -> (element=w526:dbl)  [unwired: 1 in]
        n174 = disable-structure shown="Enabled" {
          disable-tunnel: [w540 w541] -> w531
          disable-tunnel: w526 -> [w539 w542]
          frame Disabled {
            n175 = formula code="DeltaPAMB = (PAMB*0.49109778)/14.7;"("PAMB"=w539) -> ("DeltaPAMB"=w540:dbl)
          }
          frame Enabled {
            # "native LV VIs for inline VI ability"
            n176 = Multiply(x=w542, y=0.491154) -> (x*y=w541:dbl)
          }
        }
        n177 = Build Array (concatenate)(w536, "PambP" ("Param")) -> (w535:string[])
        n178 = Build Array (concatenate)(w534, w531) -> (w533:variant[])
      }
      frame 24 {
        # "DPPb\n[14.7*(PBMEAS + PBAR)/(PBAR)]-14.7"
        n179 = for {
          tunnel: w562 -> [w581]
          tunnel: w560 -> [w580]
          tunnel: w564 -> [w579]
          tunnel: w553 -> [w578]
          tunnel: [w577] -> w556 mode=indexing
          tunnel: [w576] -> w555 mode=concatenating
          tunnel: string[] ["PBMeasP", "PambP"] -> [w575] mode=indexing
          n180 = call "Get Value by Param Pattern.vi"("Default Val"=w579, "error in (no error)"=w578, "Pattern"=w575, "[Values]"=w580, "[Params]"=w581) -> ("error out"=w577:errorcluster, "[Values out]"=w576:dbl[])  [unwired: 5 in]
        }
        n181 = Merge Errors(w556) -> (w563:errorcluster)
        n182 = Index Array(array=w555) -> (element #1=w552:dbl, element #2=w551:dbl)  [unwired: 2 in]
        n183 = disable-structure shown="Enabled" {
          disable-tunnel: [w567 w568] -> w557
          disable-tunnel: w552 -> [w566 w570]
          disable-tunnel: w551 -> [w565 w569]
          frame Disabled {
            n184 = formula code="(14.7*(PBMeas + PAMB)/(PAMB))-14.7;"("PBMeas"=w566, "PAMB"=w565) -> ("DPPb"=w567:dbl)
          }
          frame Enabled {
            w574 = 14.7 ("x")
            # "native LV VIs for inline VI ability"
            n185 = Add(x=w570, y=w569) -> (x+y=w571:dbl)
            n186 = Multiply(x=w574, y=w571) -> (x*y=w572:dbl)
            n187 = Divide(x=w572, y=w569) -> (x/y=w573:dbl)
            n188 = Subtract(x=w573, y=w574) -> (x-y=w568:dbl)
          }
        }
        n189 = Build Array (concatenate)(w562, "DPPb" ("Param")) -> (w561:string[])
        n190 = Build Array (concatenate)(w560, w557) -> (w559:variant[])
      }
      frame 25 {
        # "If PBCOR is NaN, use TEGTMeas instead of calculated"
        # "Get diff between TT1AVG and table\ncolumn, then get the minimum index\nto find closest value in table"
        # "Look up columns of TT1 and PBcor and convert to DBL"
        # "TEGTcorr\nTEGTMeas - 11 (PBCOR-PBCOR-from-table)"
        n191 = Unbundle By Name(w601) -> ("RTController Data.APU Setup Info.[[CMM Table 106]]"=w599:string[][])
        n192 = call "Get CMMTable106 Clmns.vi"("Column Titles"=string[] ["TT1-Deg F", "PBCor (MIN) (PSIA)"], "[[CMM Table 106]]"=w599) -> ("Columns out"=w598:dbl[][])  [unwired: 9 in]
        n193 = Index Array(array=w598) -> (element #1=w594:dbl[], element #2=w597:dbl[])  [unwired: 4 in]
        n194 = for {
          tunnel: w609 -> [w628]
          tunnel: w607 -> [w627]
          tunnel: w586 -> [w626]
          tunnel: w596 -> [w625]
          tunnel: [w624] -> w604 mode=indexing
          tunnel: [w622] -> w603 mode=concatenating
          tunnel: string[] ["TEGTMeas", "PBCOR", "TT1AVG"] -> [w623] mode=indexing
          n195 = call "Get Value by Param Pattern.vi"("Default Val"=w626, "error in (no error)"=w625, "Pattern"=w623, "[Values]"=w627, "[Params]"=w628) -> ("error out"=w624:errorcluster, "[Values out]"=w622:dbl[])  [unwired: 5 in]
        }
        n196 = Merge Errors(w604) -> (w610:errorcluster)
        n197 = Index Array(array=w603) -> (element #1=w587:dbl, element #2=w583:dbl, element #3=w593:dbl)  [unwired: 3 in]
        n198 = Subtract(x=w593, y=w594) -> (x-y=w592:dbl[])
        n199 = Absolute Value(x=w592) -> (abs(x)=w591:dbl[])
        n200 = Array Max & Min(array=w591) -> (min index (indices)=w590:i32)  [unwired: 3 out]
        n201 = Index Array(array=w597, index=w590) -> (element=w595:dbl)
        n202 = disable-structure shown="Enabled" {
          disable-tunnel: [w614 w615] -> w589
          disable-tunnel: w587 -> [w613 w618]
          disable-tunnel: w583 -> [w612 w617]
          disable-tunnel: w595 -> [w611 w616]
          frame Disabled {
            n203 = formula code="TEGTcorr = TEGTMeas - 11*(PBCOR-PBCOR_tbl);"("TEGTMeas"=w613, "PBCOR"=w612, "PBCOR_tbl"=w611) -> ("TEGTcorr"=w614:dbl)
          }
          frame Enabled {
            # "native LV VIs for inline VI ability"
            n204 = Subtract(x=w617, y=w616) -> (x-y=w621:dbl)
            n205 = Multiply(x=11.0, y=w621) -> (x*y=w619:dbl)
            n206 = Subtract(x=w618, y=w619) -> (x-y=w615:dbl)
          }
        }
        n207 = Equal?(x=w583, y=w586) -> (x = y?=w585:bool)
        n208 = Not A Number/Path/Refnum?(number/path/refnum=w583) -> (NaN/Path/Refnum?=w582:bool)
        n209 = Or(x=w585, y=w582) -> (x .or. y?=w584:bool)
        n210 = Select(t=w587, s=w584, f=w589) -> (s? t:f=w588:dbl)
        n211 = Build Array (concatenate)(w609, "TEGTCorr" ("Param")) -> (w608:string[])
        n212 = Build Array (concatenate)(w607, w588) -> (w606:variant[])
      }
      frame 29 {
        # "HPkw\nPower *1.34102209"
        n213 = for {
          tunnel: w640 -> [w649]
          tunnel: w638 -> [w648]
          tunnel: w642 -> [w647]
          tunnel: w632 -> [w646]
          tunnel: [w645] -> w635 mode=indexing
          tunnel: [w644] -> w634 mode=concatenating
          tunnel: string[] ["Power"] -> [w643] mode=indexing
          n214 = call "Get Value by Param Pattern.vi"("Default Val"=w647, "error in (no error)"=w646, "Pattern"=w643, "[Values]"=w648, "[Params]"=w649) -> ("error out"=w645:errorcluster, "[Values out]"=w644:dbl[])  [unwired: 5 in]
        }
        n215 = Merge Errors(w635) -> (w641:errorcluster)
        n216 = Index Array(array=w634) -> (element=w631:dbl)  [unwired: 1 in]
        n217 = Multiply(x=w631, y=1.34102209) -> (x*y=w629:dbl)
        n218 = Build Array (concatenate)(w640, "HPkw" ("Param")) -> (w639:string[])
        n219 = Build Array (concatenate)(w638, w629) -> (w637:variant[])
      }
      frame 31, 32 {
        # "RPM Indicator name"
        # "N1% or N2%\n% of range\nGet Range Min and Max, subtract Min from M1 or M2 value, then divide this by range"
        n220 = Equal?(x=w658, y=31) -> (x = y?=w651:bool)
        n221 = Unbundle By Name(w675) -> ("RTController Data.APU Setup Info.[[Sensor Info]]"=w674:string[][])
        n222 = Select(t="N1" ("Pattern"), s=w651, f="ECU N2" ("Pattern")) -> (s? t:f=w654:string)
        n223 = call "Gets APU Column Index.vi"("error in (no error)"=w682, "Tag OR Name"=w654, "[Column Names]"=string[] ["Range Min", "Range Max"], "[[Array of Info]]"=w674) -> ("error out"=w671:errorcluster, "[Values out]"=w670:string[])  [unwired: 3 in, 3 out]
        n224 = Build Array(w654) -> (w672:string[])
        n225 = for {
          tunnel: w662 -> [w689]
          tunnel: w661 -> [w688]
          tunnel: w681 -> [w687]
          tunnel: w671 -> [w686]
          tunnel: [w685] -> w677 mode=indexing
          tunnel: [w684] -> w676 mode=concatenating
          tunnel: w672 -> [w683] mode=indexing
          n226 = call "Get Value by Param Pattern.vi"("Default Val"=w687, "error in (no error)"=w686, "Pattern"=w683, "[Values]"=w688, "[Params]"=w689) -> ("error out"=w685:errorcluster, "[Values out]"=w684:dbl[])  [unwired: 5 in]
        }
        n227 = Fract/Exp String To Number(string=w670) -> (number=w659:dbl[])  [unwired: 3 in, 1 out]
        n228 = Index Array(array=w659) -> (element #1=w667:dbl, element #2=w668:dbl)  [unwired: 2 in]
        n229 = Subtract(x=w668, y=w667) -> (x-y=w666:dbl)
        n230 = Merge Errors(w677) -> (w680:errorcluster)
        n231 = Index Array(array=w676) -> (element=w660:dbl)  [unwired: 1 in]
        n232 = Subtract(x=w660, y=w667) -> (x-y=w669:dbl)
        n233 = Divide(x=w669, y=w666) -> (x/y=w665:dbl)
        n234 = Multiply(x=w665, y=100.0) -> (x*y=w663:dbl)
        n235 = Select(t="N1%" ("Param"), s=w651, f="N2%" ("Param")) -> (s? t:f=w650:string)
        n236 = Build Array (concatenate)(w662, w650) -> (w679:string[])
        n237 = Build Array (concatenate)(w661, w663) -> (w678:variant[])
      }
      frame 33..38 {
        w702 = string[] ["Empty", "Empty", "Empty", "Empty", "Empty", "Empty", "Empty", "Empty", "Empty", "Empty", "Empty", "Empty", "Empty", "Empty", "Empty", "Empty", "Empty", "Empty", "Empty", "Empty", "Empty", "Empty", "Empty", "Empty", "Empty", "Empty", "Empty", "Empty", "Empty", "Empty", "Empty", "Empty", "Empty", "TPO[9,10,11,12]+", "TPO[5,6,7,8]+", "TPO[13,14,15,16]+", "TPO[13,14,15,16]+", "TPO[13,14,15,16]+", "TPO[5,6,7,8]+"]  # 30 31 32 33 34 35 36 37 38 39
        w705 = string[] ["Empty", "Empty", "Empty", "Empty", "Empty", "Empty", "Empty", "Empty", "Empty", "Empty", "Empty", "Empty", "Empty", "Empty", "Empty", "Empty", "Empty", "Empty", "Empty", "Empty", "Empty", "Empty", "Empty", "Empty", "Empty", "Empty", "Empty", "Empty", "Empty", "Empty", "Empty", "Empty", "Empty", "1-3", "1-2", "1-4", "3-4", "2-4", "2-3"]  # 30 31 32 33 34 35 36 37 38 39
        w703 = string[] ["Empty", "Empty", "Empty", "Empty", "Empty", "Empty", "Empty", "Empty", "Empty", "Empty", "Empty", "Empty", "Empty", "Empty", "Empty", "Empty", "Empty", "Empty", "Empty", "Empty", "Empty", "Empty", "Empty", "Empty", "Empty", "Empty", "Empty", "Empty", "Empty", "Empty", "Empty", "Empty", "Empty", "TPO[1,2,3,4]+", "TPO[1,2,3,4]+", "TPO[1,2,3,4]+", "TPO[5,6,7,8]+", "TPO[9,10,11,12]+", "TPO[9,10,11,12]+"]  # 30 31 32 33 34 35 36 37 38 39
        # "Note: Switched names 1-2and 1-3 when removing\nhalf of the thermocouples because quadrant\n2 and 4 no longer exist, making quadrant 3 now = 2"
        # "1-2:  33:  abs(avg(TPO1-4)-avg(TPO9-12))\n1-3:  34:  abs(avg(TPO1-4)-avg(TPO5-8))\n1-4:  35:  abs(avg(TPO1-4)-avg(TPO13-16))\n3-4:  36:  abs(avg(TPO5-8)-avg(TPO13-16))\n2-4:  37:  abs(avg(TPO9-12)-avg(TPO13-16))\n2-3:  38:  abs(avg(TPO9-12)-avg(TPO5-8))"
        # "2nd Avg Pattern"
        # "1st Avg Pattern"
        # "Splits\nFor each split, get average of each pattern"
        n238 = Index Array(array=w703, index=w690) -> (element=w700:string)
        n239 = Index Array(array=w702, index=w690) -> (element=w701:string)
        n240 = Build Array(w700, w701) -> (w699:string[])
        n241 = for {
          tunnel: w697 -> [w715]
          tunnel: w708 -> [w714]
          tunnel: w696 -> [w713]
          tunnel: [w711] -> w695 mode=indexing
          tunnel: w699 -> [w712] mode=indexing
          tunnel: w710 -> [w717]
          tunnel: [w716] -> w709 mode=indexing
          n242 = call "Get Value by Param Pattern.vi"("Default Val"=w714, "error in (no error)"=w717, "Pattern"=w712, "[Values]"=w713, "[Params]"=w715) -> ("error out"=w716:errorcluster, "[Values out]"=w718:dbl[])  [unwired: 5 in]
          n243 = call-poly <vilib>:"Mean.vi"("X"=w718) -> ("mean"=w711:dbl)  [unwired: 1 out]
        }
        n244 = Merge Errors(w709) -> (w698:errorcluster)
        n245 = Index Array(array=w695) -> (element #1=w694:dbl, element #2=w693:dbl)  [unwired: 2 in]
        n246 = Subtract(x=w694, y=w693) -> (x-y=w692:dbl)
        n247 = Absolute Value(x=w692) -> (abs(x)=w691:dbl)
        n248 = Index Array(array=w705, index=w690) -> (element=w704:string)
        n249 = Build Array (concatenate)(w697, w704) -> (w707:string[])
        n250 = Build Array (concatenate)(w696, w691) -> (w706:variant[])
      }
      frame 40 {
        # "Composite Signal Derived by Composite of Signals and a formula\n(Daniels Flow Section Formula to Be provided) Actual Bleed Air flow"
        # "P1\nPOI * 5.2"
        n251 = for {
          tunnel: w725 -> [w745]
          tunnel: w726 -> [w744]
          tunnel: w724 -> [w743]
          tunnel: w723 -> [w742]
          tunnel: [w741] -> w730 mode=indexing
          tunnel: [w740] -> w729 mode=concatenating
          tunnel: string[] ["POI"] -> [w739] mode=indexing
          n252 = call "Get Value by Param Pattern.vi"("Default Val"=w743, "error in (no error)"=w742, "Pattern"=w739, "[Values]"=w744, "[Params]"=w745) -> ("error out"=w741:errorcluster, "[Values out]"=w740:dbl[])  [unwired: 5 in]
        }
        n253 = Merge Errors(w730) -> (w722:errorcluster)
        n254 = Index Array(array=w729) -> (element=w727:dbl)  [unwired: 1 in]
        n255 = disable-structure shown="Enabled" {
          disable-tunnel: w727 -> [w735 w738]
          disable-tunnel: [w732 w736] -> w721
          frame Disabled {
            n256 = formula code="WBmeas=0;"("POI"=w735) -> ("WBmeas"=w732:dbl, "POD"=w734:dbl, "TBAD"=w733:dbl)
          }
          frame Enabled {
            # "native LV VIs for inline VI ability"
            n257 = Multiply(x=w738, y=5.2) -> (x*y=w736:dbl)
          }
        }
        n258 = Build Array (concatenate)(w725, "P1" ("Param")) -> (w720:string[])
        n259 = Build Array (concatenate)(w726, w721) -> (w719:variant[])
      }
      frame 41 {
        # "Composite Signal Derived by Composite of Signals and a formula\n(Daniels Flow Section Formula to Be provided) Actual Bleed Air flow"
        # "PODF\nPOD * 5.2"
        n260 = for {
          tunnel: w752 -> [w772]
          tunnel: w753 -> [w771]
          tunnel: w751 -> [w770]
          tunnel: w750 -> [w769]
          tunnel: [w768] -> w757 mode=indexing
          tunnel: [w767] -> w756 mode=concatenating
          tunnel: string[] ["POD"] -> [w766] mode=indexing
          n261 = call "Get Value by Param Pattern.vi"("Default Val"=w770, "error in (no error)"=w769, "Pattern"=w766, "[Values]"=w771, "[Params]"=w772) -> ("error out"=w768:errorcluster, "[Values out]"=w767:dbl[])  [unwired: 5 in]
        }
        n262 = Merge Errors(w757) -> (w749:errorcluster)
        n263 = Index Array(array=w756) -> (element=w754:dbl)  [unwired: 1 in]
        n264 = disable-structure shown="Enabled" {
          disable-tunnel: w754 -> [w762 w765]
          disable-tunnel: [w759 w763] -> w748
          frame Disabled {
            n265 = formula code="WBmeas=0;"("POI"=w762) -> ("WBmeas"=w759:dbl, "POD"=w761:dbl, "TBAD"=w760:dbl)
          }
          frame Enabled {
            # "native LV VIs for inline VI ability"
            n266 = Multiply(x=w765, y=5.2) -> (x*y=w763:dbl)
          }
        }
        n267 = Build Array (concatenate)(w752, "PODF" ("Param")) -> (w747:string[])
        n268 = Build Array (concatenate)(w753, w748) -> (w746:variant[])
      }
      frame 42 {
        # "Composite Signal Derived by Composite of Signals and a formula\n(Daniels Flow Section Formula to Be provided) Actual Bleed Air flow"
        # "P2\nP1-PODF"
        n269 = for {
          tunnel: w780 -> [w800]
          tunnel: w781 -> [w799]
          tunnel: w779 -> [w798]
          tunnel: w778 -> [w797]
          tunnel: [w796] -> w785 mode=indexing
          tunnel: [w795] -> w784 mode=concatenating
          tunnel: string[] ["P1", "PODF"] -> [w794] mode=indexing
          n270 = call "Get Value by Param Pattern.vi"("Default Val"=w798, "error in (no error)"=w797, "Pattern"=w794, "[Values]"=w799, "[Params]"=w800) -> ("error out"=w796:errorcluster, "[Values out]"=w795:dbl[])  [unwired: 5 in]
        }
        n271 = Merge Errors(w785) -> (w777:errorcluster)
        n272 = Index Array(array=w784) -> (element #1=w782:dbl, element #2=w773:dbl)  [unwired: 2 in]
        n273 = disable-structure shown="Enabled" {
          disable-tunnel: w782 -> [w790 w793]
          disable-tunnel: [w787 w791] -> w776
          disable-tunnel: w773 -> [_ w792]
          frame Disabled {
            n274 = formula code="WBmeas=0;"("POI"=w790) -> ("WBmeas"=w787:dbl, "POD"=w789:dbl, "TBAD"=w788:dbl)
          }
          frame Enabled {
            # "native LV VIs for inline VI ability"
            n275 = Subtract(x=w793, y=w792) -> (x-y=w791:dbl)
          }
        }
        n276 = Build Array (concatenate)(w780, "P2" ("Param")) -> (w775:string[])
        n277 = Build Array (concatenate)(w781, w776) -> (w774:variant[])
      }
      frame 43 {
        # "Composite Signal Derived by Composite of Signals and a formula\n(Daniels Flow Section Formula to Be provided) Actual Bleed Air flow"
        # "P1P2\nP1-P2"
        n278 = for {
          tunnel: w808 -> [w828]
          tunnel: w809 -> [w827]
          tunnel: w807 -> [w826]
          tunnel: w806 -> [w825]
          tunnel: [w824] -> w813 mode=indexing
          tunnel: [w823] -> w812 mode=concatenating
          tunnel: string[] ["P1", "P2"] -> [w822] mode=indexing
          n279 = call "Get Value by Param Pattern.vi"("Default Val"=w826, "error in (no error)"=w825, "Pattern"=w822, "[Values]"=w827, "[Params]"=w828) -> ("error out"=w824:errorcluster, "[Values out]"=w823:dbl[])  [unwired: 5 in]
        }
        n280 = Merge Errors(w813) -> (w805:errorcluster)
        n281 = Index Array(array=w812) -> (element #1=w810:dbl, element #2=w801:dbl)  [unwired: 2 in]
        n282 = disable-structure shown="Enabled" {
          disable-tunnel: w810 -> [w818 w821]
          disable-tunnel: [w815 w819] -> w804
          disable-tunnel: w801 -> [_ w820]
          frame Disabled {
            n283 = formula code="WBmeas=0;"("POI"=w818) -> ("WBmeas"=w815:dbl, "POD"=w817:dbl, "TBAD"=w816:dbl)
          }
          frame Enabled {
            # "native LV VIs for inline VI ability"
            n284 = Subtract(x=w821, y=w820) -> (x-y=w819:dbl)
          }
        }
        n285 = Build Array (concatenate)(w808, "P1P2" ("Param")) -> (w803:string[])
        n286 = Build Array (concatenate)(w809, w804) -> (w802:variant[])
      }
      frame 44 {
        # "Composite Signal Derived by Composite of Signals and a formula\n(Daniels Flow Section Formula to Be provided) Actual Bleed Air flow"
        # "RP1P2\n(P1-P2)/P1"
        n287 = for {
          tunnel: w836 -> [w856]
          tunnel: w837 -> [w855]
          tunnel: w835 -> [w854]
          tunnel: w834 -> [w853]
          tunnel: [w852] -> w841 mode=indexing
          tunnel: [w851] -> w840 mode=concatenating
          tunnel: string[] ["P1P2", "P1"] -> [w850] mode=indexing
          n288 = call "Get Value by Param Pattern.vi"("Default Val"=w854, "error in (no error)"=w853, "Pattern"=w850, "[Values]"=w855, "[Params]"=w856) -> ("error out"=w852:errorcluster, "[Values out]"=w851:dbl[])  [unwired: 5 in]
        }
        n289 = Merge Errors(w841) -> (w833:errorcluster)
        n290 = Index Array(array=w840) -> (element #1=w838:dbl, element #2=w829:dbl)  [unwired: 2 in]
        n291 = disable-structure shown="Enabled" {
          disable-tunnel: w838 -> [w846 w849]
          disable-tunnel: [w843 w847] -> w832
          disable-tunnel: w829 -> [_ w848]
          frame Disabled {
            n292 = formula code="WBmeas=0;"("POI"=w846) -> ("WBmeas"=w843:dbl, "POD"=w845:dbl, "TBAD"=w844:dbl)
          }
          frame Enabled {
            # "native LV VIs for inline VI ability"
            n293 = Divide(x=w849, y=w848) -> (x/y=w847:dbl)
          }
        }
        n294 = Build Array (concatenate)(w836, "RP1P2" ("Param")) -> (w831:string[])
        n295 = Build Array (concatenate)(w837, w832) -> (w830:variant[])
      }
      frame 45 {
        # "native LV VIs for inline VI ability"
        # "Composite Signal Derived by Composite of Signals and a formula\n(Daniels Flow Section Formula to Be provided) Actual Bleed Air flow"
        # "Y1 \nThree cases -see below"
        n296 = for {
          tunnel: w864 -> [w900]
          tunnel: w865 -> [w899]
          tunnel: w863 -> [w898]
          tunnel: w862 -> [w897]
          tunnel: [w896] -> w869 mode=indexing
          tunnel: [w895] -> w868 mode=concatenating
          tunnel: string[] ["DO", "RP1P2"] -> [w894] mode=indexing
          n297 = call "Get Value by Param Pattern.vi"("Default Val"=w898, "error in (no error)"=w897, "Pattern"=w894, "[Values]"=w899, "[Params]"=w900) -> ("error out"=w896:errorcluster, "[Values out]"=w895:dbl[])  [unwired: 5 in]
        }
        n298 = Merge Errors(w869) -> (w861:errorcluster)
        n299 = Index Array(array=w868) -> (element #1=w866:dbl, element #2=w857:dbl)  [unwired: 2 in]
        n300 = disable-structure shown="Enabled" {
          disable-tunnel: w866 -> [w874 w878]
          disable-tunnel: [w871 w875] -> w860
          disable-tunnel: w857 -> [_ w876]
          frame Disabled {
            n301 = formula code="WBmeas=0;"("POI"=w874) -> ("WBmeas"=w871:dbl, "POD"=w873:dbl, "TBAD"=w872:dbl)
          }
          frame Enabled {
            n302 = Number To Decimal String(number=w878) -> (decimal integer string=w877:string)  [unwired: 1 in]
            n303 = case shown="\"5\"" w877 {
              tunnel: w876 -> [w880 w885 w892]
              tunnel: [w879 w884 w889] -> w875
              frame "3.025", Default {
                n304 = Multiply(x=-0.2991 ("Default Val"), y=w880) -> (x*y=w882:dbl)
                n305 = Add(x=w882, y=1.0006) -> (x+y=w879:dbl)
              }
              frame "4" {
                n306 = Multiply(x=-0.305 ("Default Val"), y=w885) -> (x*y=w887:dbl)
                n307 = Add(x=w887, y=1.0008) -> (x+y=w884:dbl)
              }
              frame "5" {
                n308 = Multiply(x=-0.318 ("Default Val"), y=w892) -> (x*y=w891:dbl)
                n309 = Add(x=w891, y=1.001) -> (x+y=w889:dbl)
              }
            }
          }
        }
        n310 = Build Array (concatenate)(w864, "Y1" ("Param")) -> (w859:string[])
        n311 = Build Array (concatenate)(w865, w860) -> (w858:variant[])
      }
      frame 46 {
        # "native LV VIs for inline VI ability"
        # "Composite Signal Derived by Composite of Signals and a formula\n(Daniels Flow Section Formula to Be provided) Actual Bleed Air flow"
        # "A \nA = K(2*gc/R)^0.5"
        n312 = for {
          tunnel: w907 -> [w932]
          tunnel: w908 -> [w931]
          tunnel: w906 -> [w930]
          tunnel: w905 -> [w929]
          tunnel: [w928] -> w912 mode=indexing
          tunnel: [w927] -> w911 mode=concatenating
          tunnel: string[] ["K"] -> [w926] mode=indexing
          n313 = call "Get Value by Param Pattern.vi"("Default Val"=w930, "error in (no error)"=w929, "Pattern"=w926, "[Values]"=w931, "[Params]"=w932) -> ("error out"=w928:errorcluster, "[Values out]"=w927:dbl[])  [unwired: 5 in]
        }
        n314 = Merge Errors(w912) -> (w904:errorcluster)
        n315 = Index Array(array=w911) -> (element=w909:dbl)  [unwired: 1 in]
        n316 = disable-structure shown="Enabled" {
          disable-tunnel: w909 -> [w917 w919]
          disable-tunnel: [w914 w918] -> w903
          frame Disabled {
            n317 = formula code="WBmeas=0;"("POI"=w917) -> ("WBmeas"=w914:dbl, "POD"=w916:dbl, "TBAD"=w915:dbl)
          }
          frame Enabled {
            n318 = Multiply(x=2.0, y=32.1442095) -> (x*y=w923:dbl)
            n319 = Divide(x=w923, y=53.35) -> (x/y=w921:dbl)
            n320 = Square Root(x=w921) -> (sqrt(x)=w920:dbl)
            n321 = Multiply(x=w920, y=w919) -> (x*y=w918:dbl)
          }
        }
        n322 = Build Array (concatenate)(w907, "A" ("Param")) -> (w902:string[])
        n323 = Build Array (concatenate)(w908, w903) -> (w901:variant[])
      }
      frame 47 {
        # "native LV VIs for inline VI ability"
        # "Composite Signal Derived by Composite of Signals and a formula\n(Daniels Flow Section Formula to Be provided) Actual Bleed Air flow"
        # "B \nB = Y1(1-(P2/P1))0.5 ="
        n324 = for {
          tunnel: w941 -> [w966]
          tunnel: w942 -> [w965]
          tunnel: w940 -> [w964]
          tunnel: w939 -> [w963]
          tunnel: [w962] -> w946 mode=indexing
          tunnel: [w961] -> w945 mode=concatenating
          tunnel: string[] ["Y1", "P2", "P1"] -> [w960] mode=indexing
          n325 = call "Get Value by Param Pattern.vi"("Default Val"=w964, "error in (no error)"=w963, "Pattern"=w960, "[Values]"=w965, "[Params]"=w966) -> ("error out"=w962:errorcluster, "[Values out]"=w961:dbl[])  [unwired: 5 in]
        }
        n326 = Merge Errors(w946) -> (w938:errorcluster)
        n327 = Index Array(array=w945) -> (element #1=w943:dbl, element #2=w934:dbl, element #3=w933:dbl)  [unwired: 3 in]
        n328 = disable-structure shown="Enabled" {
          disable-tunnel: w943 -> [w951 w958]
          disable-tunnel: [w948 w957] -> w937
          disable-tunnel: w934 -> [_ w955]
          disable-tunnel: w933 -> [_ w954]
          frame Disabled {
            n329 = formula code="WBmeas=0;"("POI"=w951) -> ("WBmeas"=w948:dbl, "POD"=w950:dbl, "TBAD"=w949:dbl)
          }
          frame Enabled {
            n330 = Divide(x=w955, y=w954) -> (x/y=w953:dbl)
            n331 = Subtract(x=1.0, y=w953) -> (x-y=w952:dbl)
            n332 = Square Root(x=w952) -> (sqrt(x)=w959:dbl)
            n333 = Multiply(x=w959, y=w958) -> (x*y=w957:dbl)
          }
        }
        n334 = Build Array (concatenate)(w941, "B" ("Param")) -> (w936:string[])
        n335 = Build Array (concatenate)(w942, w937) -> (w935:variant[])
      }
      frame 48 {
        # "=3.14*(G15^2)/4"
        # "native LV VIs for inline VI ability"
        # "Composite Signal Derived by Composite of Signals and a formula\n(Daniels Flow Section Formula to Be provided) Actual Bleed Air flow"
        # "C \nC = (Tbmeas)0.5/P1*A ="
        n336 = for {
          tunnel: w975 -> [w1005]
          tunnel: w976 -> [w1004]
          tunnel: w974 -> [w1003]
          tunnel: w973 -> [w1002]
          tunnel: [w1001] -> w980 mode=indexing
          tunnel: [w1000] -> w979 mode=concatenating
          tunnel: string[] ["TBMeas", "P1", "DO"] -> [w999] mode=indexing
          n337 = call "Get Value by Param Pattern.vi"("Default Val"=w1003, "error in (no error)"=w1002, "Pattern"=w999, "[Values]"=w1004, "[Params]"=w1005) -> ("error out"=w1001:errorcluster, "[Values out]"=w1000:dbl[])  [unwired: 5 in]
        }
        n338 = Merge Errors(w980) -> (w972:errorcluster)
        n339 = Index Array(array=w979) -> (element #1=w977:dbl, element #2=w968:dbl, element #3=w967:dbl)  [unwired: 3 in]
        n340 = disable-structure shown="Enabled" {
          disable-tunnel: w977 -> [w985 w998]
          disable-tunnel: [w982 w986] -> w971
          disable-tunnel: w968 -> [_ w989]
          disable-tunnel: w967 -> [_ w996]
          frame Disabled {
            n341 = formula code="WBmeas=0;"("POI"=w985) -> ("WBmeas"=w982:dbl, "POD"=w984:dbl, "TBAD"=w983:dbl)
          }
          frame Enabled {
            n342 = Square Root(x=w998) -> (sqrt(x)=w988:dbl)
            n343 = Square(x=w996) -> (x^2=w995:dbl)
            n344 = Multiply(x=w995, y=3.141592653589793) -> (x*y=w994:dbl)
            n345 = Divide(x=w994, y=4.0) -> (x/y=w992:dbl)
            n346 = Multiply(x=144.0, y=w992) -> (x*y=w990:dbl)
            n347 = Multiply(x=w989, y=w990) -> (x*y=w987:dbl)
            n348 = Divide(x=w988, y=w987) -> (x/y=w986:dbl)
          }
        }
        n349 = Build Array (concatenate)(w975, "B" ("Param")) -> (w970:string[])
        n350 = Build Array (concatenate)(w976, w971) -> (w969:variant[])
      }
      frame 49 {
        # "=3.14*(G15^2)/4"
        # "native LV VIs for inline VI ability"
        # "Composite Signal Derived by Composite of Signals and a formula\n(Daniels Flow Section Formula to Be provided) Actual Bleed Air flow"
        # "WBmeas \n(A*B)/C"
        n351 = for {
          tunnel: w1014 -> [w1036]
          tunnel: w1015 -> [w1035]
          tunnel: w1013 -> [w1034]
          tunnel: w1012 -> [w1033]
          tunnel: [w1032] -> w1019 mode=indexing
          tunnel: [w1031] -> w1018 mode=concatenating
          tunnel: string[] ["A", "B", "C"] -> [w1030] mode=indexing
          n352 = call "Get Value by Param Pattern.vi"("Default Val"=w1034, "error in (no error)"=w1033, "Pattern"=w1030, "[Values]"=w1035, "[Params]"=w1036) -> ("error out"=w1032:errorcluster, "[Values out]"=w1031:dbl[])  [unwired: 5 in]
        }
        n353 = Merge Errors(w1019) -> (w1011:errorcluster)
        n354 = Index Array(array=w1018) -> (element #1=w1016:dbl, element #2=w1007:dbl, element #3=w1006:dbl)  [unwired: 3 in]
        n355 = disable-structure shown="Enabled" {
          disable-tunnel: w1016 -> [w1024 w1029]
          disable-tunnel: [w1021 w1025] -> w1010
          disable-tunnel: w1007 -> [_ w1028]
          disable-tunnel: w1006 -> [_ w1026]
          frame Disabled {
            n356 = formula code="WBmeas=0;"("POI"=w1024) -> ("WBmeas"=w1021:dbl, "POD"=w1023:dbl, "TBAD"=w1022:dbl)
          }
          frame Enabled {
            n357 = Multiply(x=w1029, y=w1028) -> (x*y=w1027:dbl)
            n358 = Divide(x=w1027, y=w1026) -> (x/y=w1025:dbl)
          }
        }
        n359 = Build Array (concatenate)(w1014, "WBmeas" ("Param")) -> (w1009:string[])
        n360 = Build Array (concatenate)(w1015, w1010) -> (w1008:variant[])
      }
      frame 50 {
        # "native LV VIs for inline VI ability"
        # "Composite Signal Derived by Composite of Signals and a formula\n(Daniels Flow Section Formula to Be provided) Actual Bleed Air flow"
        # "WBcor \nWBCOR = WBMEAS/dPAMB"
        n361 = for {
          tunnel: w1044 -> [w1064]
          tunnel: w1045 -> [w1063]
          tunnel: w1043 -> [w1062]
          tunnel: w1042 -> [w1061]
          tunnel: [w1060] -> w1049 mode=indexing
          tunnel: [w1059] -> w1048 mode=concatenating
          tunnel: string[] ["WBmeas", "DeltaPAMB1"] -> [w1058] mode=indexing
          n362 = call "Get Value by Param Pattern.vi"("Default Val"=w1062, "error in (no error)"=w1061, "Pattern"=w1058, "[Values]"=w1063, "[Params]"=w1064) -> ("error out"=w1060:errorcluster, "[Values out]"=w1059:dbl[])  [unwired: 5 in]
        }
        n363 = Merge Errors(w1049) -> (w1041:errorcluster)
        n364 = Index Array(array=w1048) -> (element #1=w1046:dbl, element #2=w1037:dbl)  [unwired: 2 in]
        n365 = disable-structure shown="Enabled" {
          disable-tunnel: w1046 -> [w1054 w1056]
          disable-tunnel: [w1051 w1057] -> w1040
          disable-tunnel: w1037 -> [_ w1055]
          frame Disabled {
            n366 = formula code="WBmeas=0;"("POI"=w1054) -> ("WBmeas"=w1051:dbl, "POD"=w1053:dbl, "TBAD"=w1052:dbl)
          }
          frame Enabled {
            n367 = Divide(x=w1056, y=w1055) -> (x/y=w1057:dbl)
          }
        }
        n368 = Build Array (concatenate)(w1044, "WBcor" ("Param")) -> (w1039:string[])
        n369 = Build Array (concatenate)(w1045, w1040) -> (w1038:variant[])
      }
      frame 51 {
        # "native LV VIs for inline VI ability"
        # "Composite Signal Derived by Composite of Signals and a formula\n(Daniels Flow Section Formula to Be provided) Actual Bleed Air flow"
        # "DCF \nWBmeas*((qB)^0.5)/dB"
        n370 = for {
          tunnel: w1072 -> [w1093]
          tunnel: w1073 -> [w1092]
          tunnel: w1071 -> [w1091]
          tunnel: w1070 -> [w1090]
          tunnel: [w1089] -> w1077 mode=indexing
          tunnel: [w1088] -> w1076 mode=concatenating
          tunnel: string[] ["ThetaB", "DeltaB"] -> [w1087] mode=indexing
          n371 = call "Get Value by Param Pattern.vi"("Default Val"=w1091, "error in (no error)"=w1090, "Pattern"=w1087, "[Values]"=w1092, "[Params]"=w1093) -> ("error out"=w1089:errorcluster, "[Values out]"=w1088:dbl[])  [unwired: 5 in]
        }
        n372 = Merge Errors(w1077) -> (w1069:errorcluster)
        n373 = Index Array(array=w1076) -> (element #1=w1074:dbl, element #2=w1065:dbl)  [unwired: 2 in]
        n374 = disable-structure shown="Enabled" {
          disable-tunnel: w1074 -> [w1082 w1084]
          disable-tunnel: [w1079 w1086] -> w1068
          disable-tunnel: w1065 -> [_ w1085]
          frame Disabled {
            n375 = formula code="WBmeas=0;"("POI"=w1082) -> ("WBmeas"=w1079:dbl, "POD"=w1081:dbl, "TBAD"=w1080:dbl)
          }
          frame Enabled {
            n376 = Square Root(x=w1084) -> (sqrt(x)=w1083:dbl)
            n377 = Divide(x=w1083, y=w1085) -> (x/y=w1086:dbl)
          }
        }
        n378 = Build Array (concatenate)(w1072, "WBcor" ("Param")) -> (w1067:string[])
        n379 = Build Array (concatenate)(w1073, w1068) -> (w1066:variant[])
      }
    }
    n380 = Equal?(x=dbl[] [inf, -inf, -404.0], y=w90) -> (x = y?=w93:bool[])
    n381 = Or Array Elements(Boolean array=w93) -> (logical OR=w92:bool)
    n382 = Select(t=w91, s=w92, f=w90) -> (s? t:f=w89:dbl)
  }
  n383 = feedback-in #1(w20) -> ()
  n384 = feedback #1() -> (w19:bool)  [unwired: 1 in]
  n385 = Not(x=w19) -> (.not. x?=w18:bool)
  n386 = And(x=w20, y=w18) -> (x .and. y?=w22:bool)
  n387 = case shown="True" w22 {
    frame False {
    }
    frame True {
      # "If fault, run this subvi, get new calc indices order array. \nMove new contant to this subvi"
      # "Alert developer if changes\noccur to Calc Data cluster,\nbut they forget to update\nthe indices array using\nthe VI in utilities"
      n388 = call "Error.vi"("Error"=errorcluster {"status"=TRUE, "code"=-1234, "source"="Calculated Values Cluster size mismatch with Indices Array"}) -> ()  [unwired: 10 in, 1 out]
      n389 = call "Generate Calc Indices Array.vi"() -> ()  [unwired: 12 in]
    }
  }
  n390 = call-poly <userlib>:"Reorder Array2__ogtk.vi"("indices"=w2, "array"=w5) -> ("reordered array"=w4:dbl[])  [unwired: 9 in]
  n391 = Index Array(array=w4) -> (element #1=w79:dbl, element #2=w78:dbl, element #3=w77:dbl, element #4=w76:dbl, element #5=w75:dbl, element #6=w74:dbl, element #7=w73:dbl, element #8=w72:dbl, element #9=w71:dbl, element #10=w70:dbl, element #11=w69:dbl, element #12=w68:dbl, element #13=w67:dbl, element #14=w66:dbl, element #15=w65:dbl, element #16=w64:dbl, element #17=w63:dbl, element #18=w62:dbl, element #19=w61:dbl, element #20=w60:dbl, element #21=w59:dbl, element #22=w58:dbl, element #23=w57:dbl, element #24=w56:dbl, element #25=w55:dbl, element #26=w54:dbl, element #27=w53:dbl, element #28=w52:dbl, element #29=w51:dbl, element #30=w50:dbl, element #31=w49:dbl, element #32=w48:dbl, element #33=w47:dbl, element #34=w46:dbl, element #35=w45:dbl, element #36=w44:dbl, element #37=w43:dbl, element #38=w42:dbl, element #39=w41:dbl, element #40=w40:dbl, element #41=w39:dbl, element #42=w38:dbl, element #43=w37:dbl, element #44=w36:dbl, element #45=w35:dbl, element #46=w34:dbl, element #47=w33:dbl, element #48=w32:dbl, element #49=w15:dbl, element #50=w14:dbl, element #51=w13:dbl, element #52=w12:dbl, element #53=w11:dbl, element #54=w10:dbl, element #55=w9:dbl, element #56=w8:dbl)  [unwired: 56 in]
  n392 = Merge Errors(w31) -> (→"error out":errorcluster)
  n393 = Bundle(cluster=T16 {"C.00"=0.0, "C.01"=0.0, "C.02"=0.0, "C.03"=0.0, "C.04"=0.0, "C.05"=0.0, "C.06"=0.0, "C.07"=0.0, "C.08"=0.0, "C.09"=0.0, "C.10"=0.0, "C.11"=0.0, "C.12"=0.0, "C.13"=0.0, "C.14"=0.0, "C.15"=0.0, "C.16"=0.0, "C.17"=0.0, "C.18"=0.0, "C.19"=0.0, "C.20"=0.0, "C.21"=0.0, "C.22"=0.0, "C.23"=0.0, "C.24"=0.0, "C.25"=0.0, "C.26"=0.0, "C.27"=0.0, "C.28"=0.0, "C.29"=0.0, "C.30"=0.0, "C.31"=0.0, "C.32"=0.0, "C.33"=0.0, "C.34"=0.0, "C.35"=0.0, "C.36"=0.0, "C.37"=0.0, "C.38"=0.0, "C.39"=0.0, "C.40"=0.0, "C.41"=0.0, "C.42"=0.0, "C.43"=0.0, "C.44"=0.0, "C.45"=0.0, "C.46"=0.0, "C.47"=0.0, "C.48"=0.0, "C.49"=0.0, "C.50"=0.0, "C.51"=0.0, "C.52"=0.0, "C.53"=0.0, "C.54"=0.0, "C.56"=0.0} ("Calculated Values out"), "C.00"=w79, "C.01"=w78, "C.02"=w77, "C.03"=w76, "C.04"=w75, "C.05"=w74, "C.06"=w73, "C.07"=w72, "C.08"=w71, "C.09"=w70, "C.10"=w69, "C.11"=w68, "C.12"=w67, "C.13"=w66, "C.14"=w65, "C.15"=w64, "C.16"=w63, "C.17"=w62, "C.18"=w61, "C.19"=w60, "C.20"=w59, "C.21"=w58, "C.22"=w57, "C.23"=w56, "C.24"=w55, "C.25"=w54, "C.26"=w53, "C.27"=w52, "C.28"=w51, "C.29"=w50, "C.30"=w49, "C.31"=w48, "C.32"=w47, "C.33"=w46, "C.34"=w45, "C.35"=w44, "C.36"=w43, "C.37"=w42, "C.38"=w41, "C.39"=w40, "C.40"=w39, "C.41"=w38, "C.42"=w37, "C.43"=w36, "C.44"=w35, "C.45"=w34, "C.46"=w33, "C.47"=w32, "C.48"=w15, "C.49"=w14, "C.50"=w13, "C.51"=w12, "C.52"=w11, "C.53"=w10, "C.54"=w9, "C.56"=w8) -> (→"Calculated Values out":T16)
